vi "PositionSave_MD.vi"() -> ()   [LabVIEW 2012]
doc: "<b>Description</b>\n-------------\nThis is the Main VI for the Position Save Module and has a UI.\n\nThe module has a dependency with the main Sci-Scan software as it listens for events using the GFG."
uses:
  Custom Control and Typedefs/ChannelSelector_for_PosSave.ctl
  Custom Controls/PositionSaveMod.ctl
  Custom Control and Typedefs/Overlay Control.ctl
  SubVIs/PositionSaveFGVCommands.ctl
  Custom Control and Typedefs/UI Controls Refnum.ctl
  <vilib>/vision/Image Controls.llb/IMAQ Image.ctl
  Custom Control and Typedefs/ImageCluster.ctl
  SubVIs/Chnl_2_tab_Commands.ctl
  SubVIs/Image Validity FGV_Commands.ctl
  Custom Controls/MAIN Image panel tab Control type def.ctl
  CommonResource VIs/UI Control and Indicator properties_Commands.ctl
  CommonResource VIs/FormatTableStyle_Commands.ctl
  Custom Control and Typedefs/PositionData.ctl
  SubVIs/ImageIO_commands.ctl
  GFG/GFG library.lvlib
panel:
  in  "FOCUS2":bool
  in  "Overlay Controls":T1={"auto scale\n      Red "=TRUE, "Min Max Saved (Green)"={0.0, 1618.0}, "auto scale\n      Green"=TRUE, "Min Max Saved (Red)"={0.0, 1618.0}} {"Min Max Saved (Red)" scale=-100.0..2047.0; "Min Max Saved (Green)" scale=-100.0..2047.0}
  in  "Hide":T2
  in  "Copy Button":bool
  out "File Path":path
  in  "Overlay":bool
  in  "Table Navigation Cluster":T3
  in  "Vert_Cluster":T4
  in  "Big_Table":string[][](table)
  in  "Notes_Table":string[][](table)
  in  "Source":T5
  in  "step.size.z 2":u16(ring)=6 items=["  1"=1, "  2"=2, "  5"=5, " 10"=10, " 20"=20, " 50"=50, "100"=100]
  in  "Stage Stop 2":bool
  in  "Z UP 2":bool
  in  "Z DOWN 2":bool
  out "String 26":string
  in  "step.size.xy 2":u16(ring)=6 items=["  1"=1, "  2"=2, "  5"=5, " 10"=10, " 20"=20, " 50"=50, "100"=100]
  in  "Y UP 2":bool
  in  "X LEFT 2":bool
  in  "Y DOWN 2":bool
  in  "X RIGHT 2":bool
  out "String 25":string
  in  "setY 2":dbl caption="Z-Stepper" format="%#.1f"
  in  "setX 2":dbl caption="Z-Stepper" format="%#.1f"
  in  "setZ 2":dbl caption="set" format="%#.1f"
  out "String 24":string
  out "posZ 2":dbl caption="actual" format="%#.1f"
  out "posX 2":dbl caption="Z-Stepper" format="%#.1f"
  out "posY 2":dbl caption="Z-Stepper" format="%#.1f"
  out "String 23":string
  in  "Hor_Cluster":T6
  out "XY Graph":cluster{dbl[], dbl[]}[](graph)
  out "Saved Image":T7(plugin-control)
  out "Current Image":T7(plugin-control)
  # "current pos."
  # "go to pos."
  # "Red (Current Image)"
  # "Green (Saved Image)"
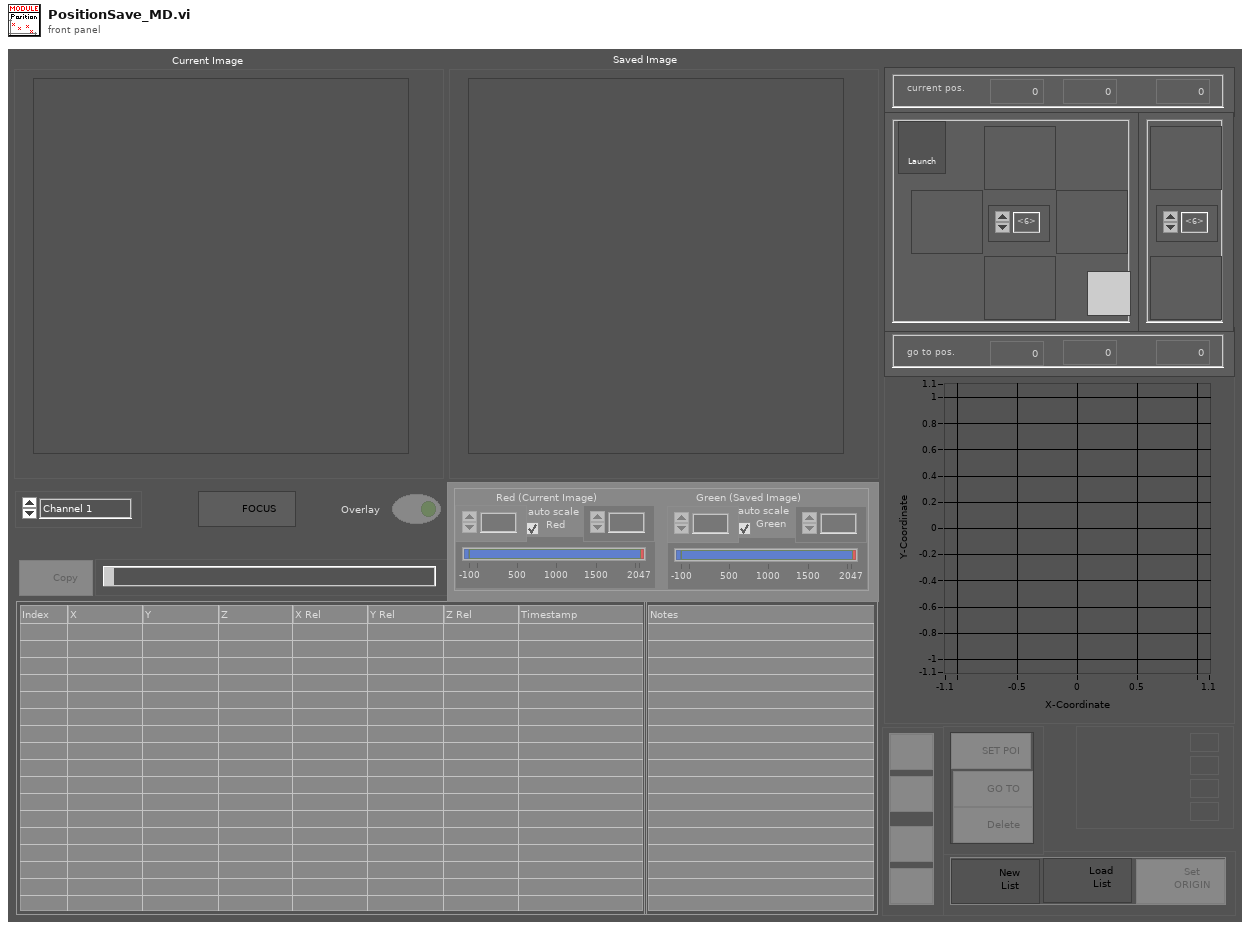
[diagram p1: front panel]
types:
  T1 = typedef "Overlay Control.ctl" = cluster{"auto scale\n      Red ":bool, "Min Max Saved (Green)":cluster{dbl, dbl}, "auto scale\n      Green":bool, "Min Max Saved (Red)":cluster{dbl, dbl}}
  T2 = typedef "PositionSaveMod.ctl" = bool
  T3 = cluster{"Table Index Up":bool, "Table Index Up-End":bool, "Table Index Down":bool, "Table Index Down-End":bool}
  T4 = cluster{"Delete item":bool, "SET POI":bool, "GO TO":bool}
  T5 = typedef "ChannelSelector_for_PosSave.ctl" = enum16{"Channel 1", "Channel 2", "Channel 3", "Channel 4"}
  T6 = cluster{"New List":bool, "Load List":bool, "Set new Origin":bool}
  T7 = typedef "IMAQ Image.ctl" = refnum<image>
  T8 = typedef "Image Type" = u32
  T9 = typedef "UI Controls Refnum.ctl" = cluster{"GO TO":refnum<vi>, "Load List":refnum<vi>, "Big Table":refnum<vi>, "Notes Table":refnum<vi>, "New List":refnum<vi>, "Delete Item":refnum<vi>, "Set New Origin":refnum<vi>, "Set POI":refnum<vi>, "Saved Image":refnum<vi>, "Current Image":refnum<vi>, "step.size.xy 2":refnum<vi>, "step.size.z 2":refnum<vi>, "Source":refnum<vi>, "Table Up-End":refnum<vi>, "Table Up":refnum<vi>, "Table Down":refnum<vi>, "Table Down-End":refnum<vi>, "Copy Button":refnum<vi>, "Hide":refnum<vi>, "Overlay Controls":refnum<vi>, "Overlay":refnum<vi>, "XYGraph":refnum<vi>, "FOCUS2":refnum<vi>}
  T10 = typedef "PositionSaveFGVCommands.ctl" = enum16{"Initialize", "NewList", "LoadList", "CopyList", "DeleteSelected", "SetPosition", "SetNewOrigin", "UpdateEntireTable", "GetPosition", "Shutdown and Cleanup"}
  T11 = typedef "ImageCluster.ctl" = cluster{"CurrentImage":T7, "SavedImage":T7}
  T12 = enum32{"Invalid", "Standard", "Closed", "Hidden", "Minimized", "Maximized"}
  T13 = typedef "Image Validity FGV_Commands.ctl" = enum16{"Set validity status", "Get Validity status"}
  T14 = typedef "Chnl_2_tab_Commands.ctl" = enum16{"ChannelToTab", "TabToChannel"}
  T15 = typedef "UI Control and Indicator properties_Commands.ctl" = enum16{"Enable", "Disable", "Disable and Grey", "Make Visible", "Make Invisible"}
  T16 = typedef "MAIN Image panel tab Control type def.ctl" = enum32{"Channel 1", "Channel 2", "Channel 3", "Channel 4", "all channels", "RGB overlay", "ROI", "arbitrary line scan"}
  T17 = cluster{"moveXabs":dbl, "moveYabs":dbl, "moveZabs":dbl}
  T18 = typedef "FormatTableStyle_Commands.ctl" = enum16{"Colour Row", "Uncolour Row", "Bold Row", "Clear table", "UpdateVisibleRows"}
  T19 = typedef "PositionData.ctl" = cluster{"X":dbl, "Y":dbl, "Z":dbl, "Base Path":path}
  T20 = typedef "ImageIO_commands.ctl" = enum16{"ReadImage", "WriteImage"}
  T21 = cluster{"WaveformChartRef":refnum<vi>, "DigitalRef":refnum<vi>, "ArrayRef":refnum<vi>, "TabControlRef":refnum<vi>, "EnumRef":refnum<vi>, "RingRef":refnum<vi>, "BooleanRef":refnum<vi>, "KnobRef":refnum<vi>, "SlideRef":refnum<vi>, "PathRef":refnum<vi>, "StringRef":refnum<vi>, "ComboBox":refnum<vi>, "WaveformGraphRef":refnum<vi>}
  T22 = typedef "LVRowAndColumnTypeDef.ctl" = cluster{"Row":i32, "Column":i32}
  T23 = typedef "eventvkey.ctl" = enum16{"ASCII", "Enter", "Return", "Shift", "Ctrl", "Alt", "Cmd", "Opt", "Caps", "NumLock", "Clear", "Break", "Up", "Down", "Left", "Right", "Insert", "Delete", "Home", "End", "PageUp", "PageDown", "Escape", "Help", "Pause", "ScrollLock", "F1", "F2", "F3", "F4", "F5", "F6", "F7", "F8", "F9", "F10", "F11", "F12", "F13", "F14", "F15", "F16", "F17", "F18", "F19", "F20", "F21", "F22", "F23", "F24", "Play", "VolumeUp", "VolumeDown", "Mute", "Two Byte Char"}
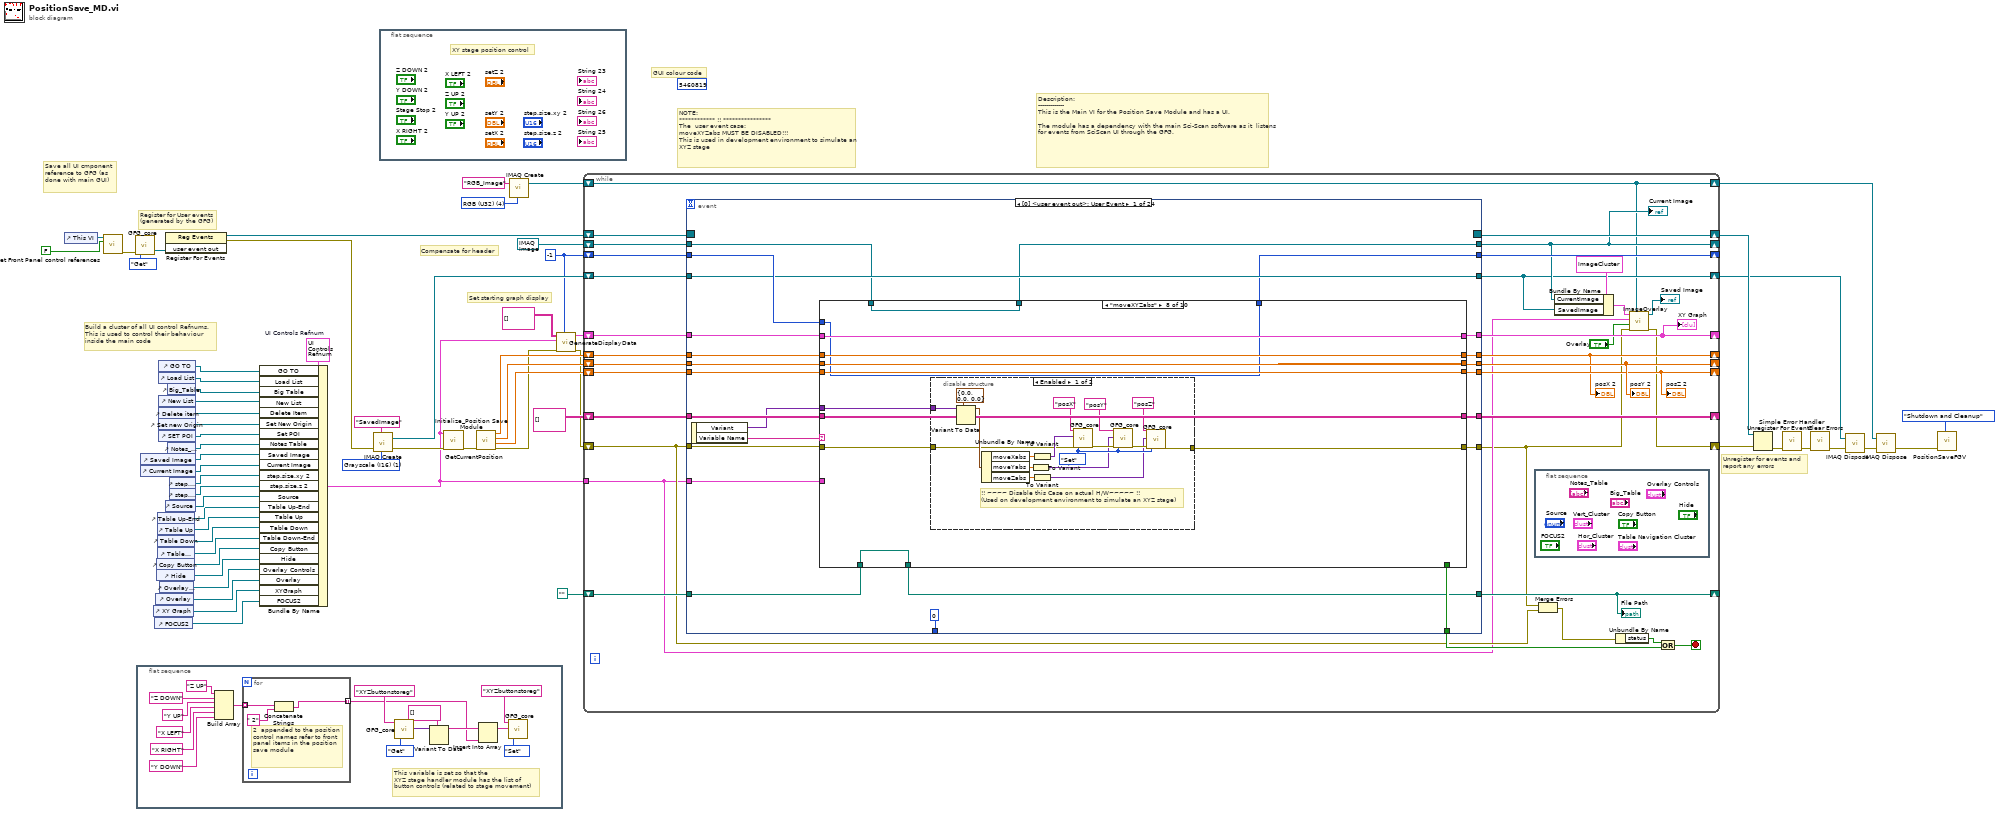
[diagram p0: block diagram]
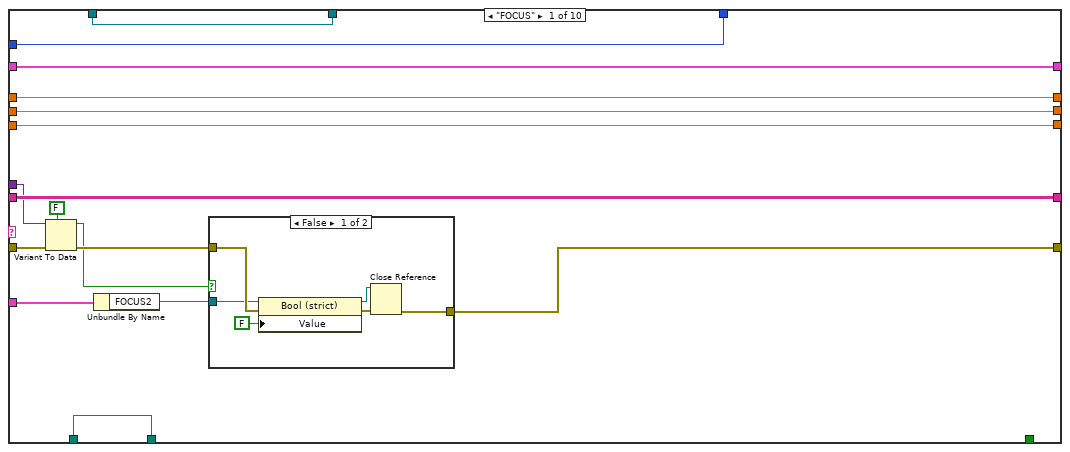
[diagram p2: hidden frame]
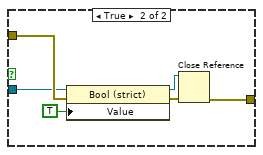
[diagram p3: hidden frame]
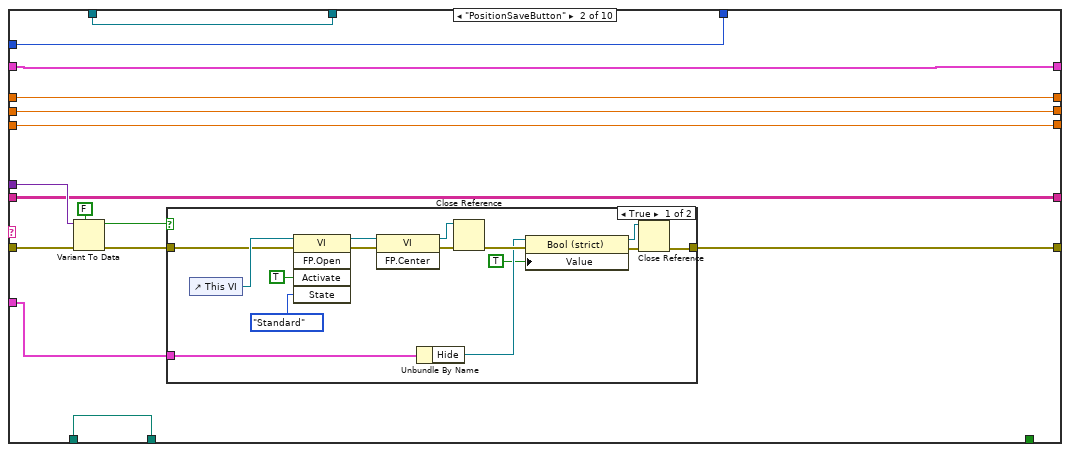
[diagram p4: hidden frame]
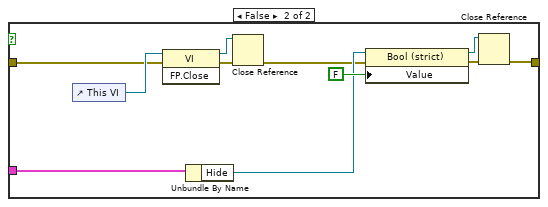
[diagram p5: hidden frame]
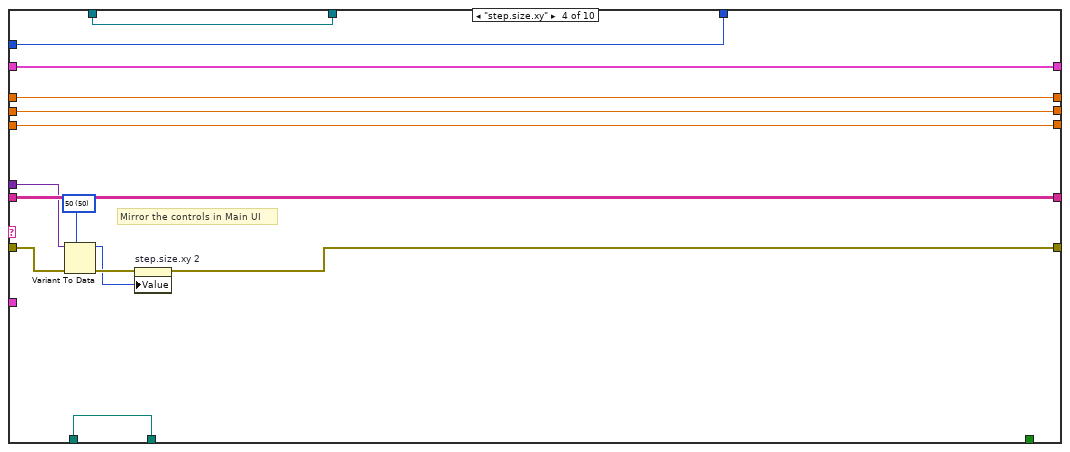
[diagram p7: hidden frame]
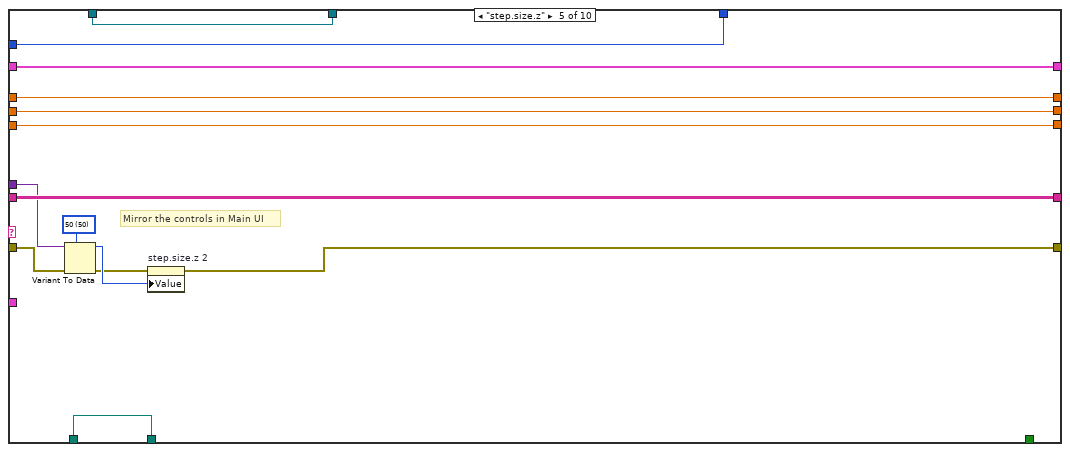
[diagram p8: hidden frame]
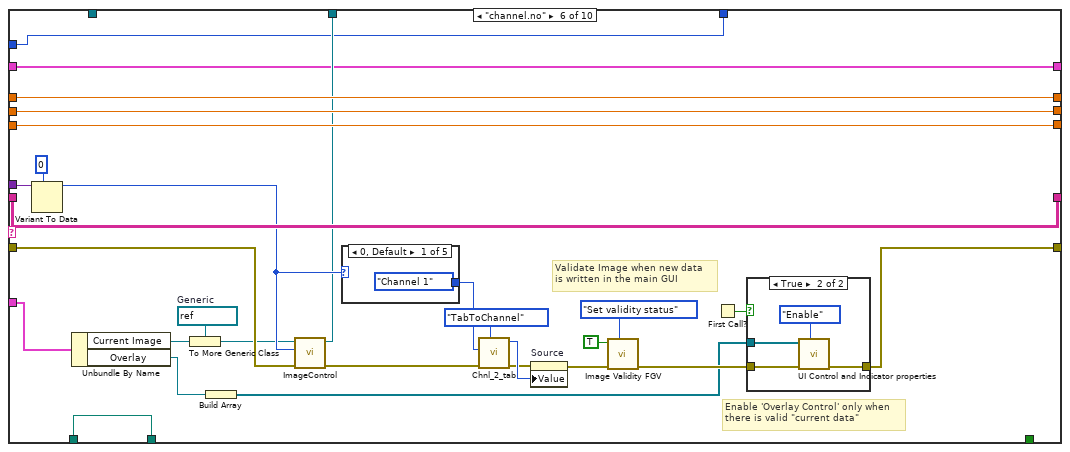
[diagram p9: hidden frame]
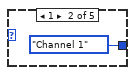
[diagram p11: hidden frame]
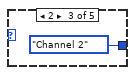
[diagram p12: hidden frame]
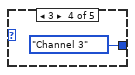
[diagram p13: hidden frame]
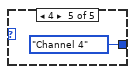
[diagram p14: hidden frame]
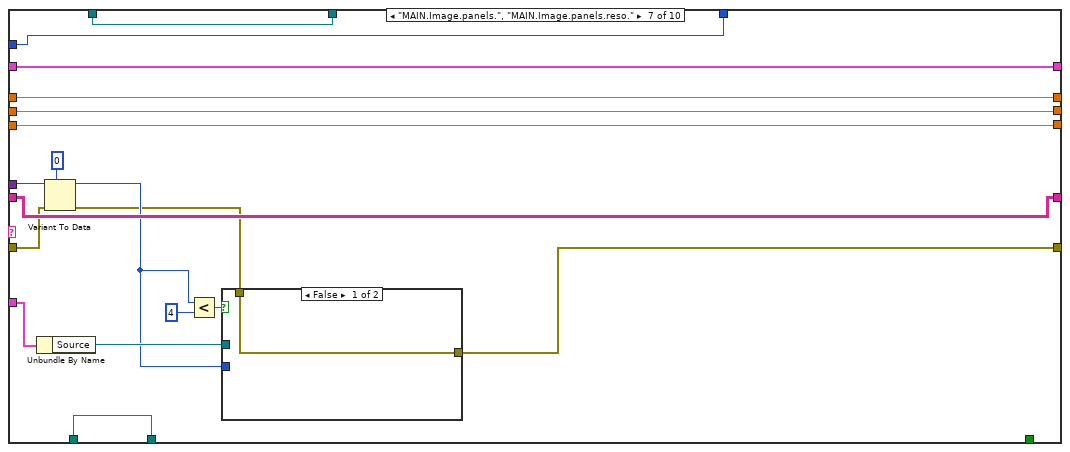
[diagram p15: hidden frame]
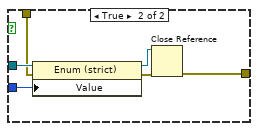
[diagram p16: hidden frame]
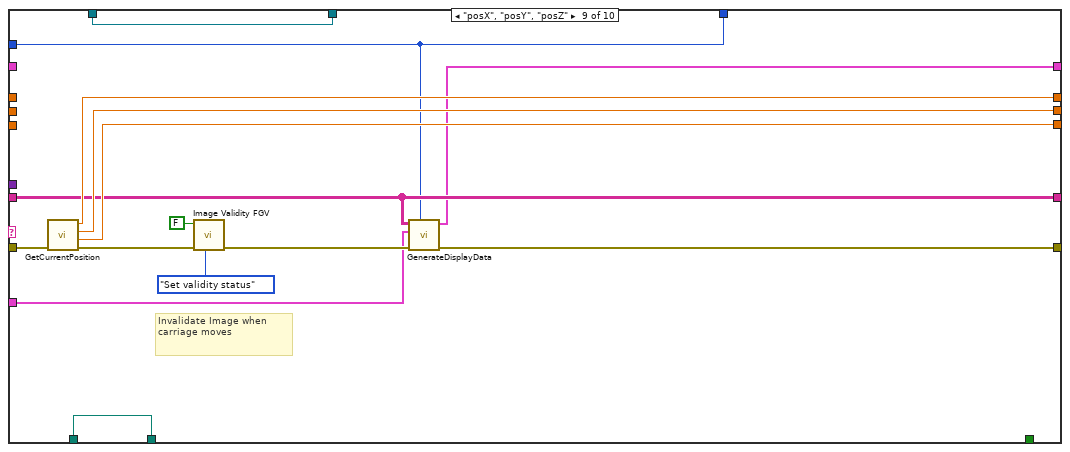
[diagram p18: hidden frame]
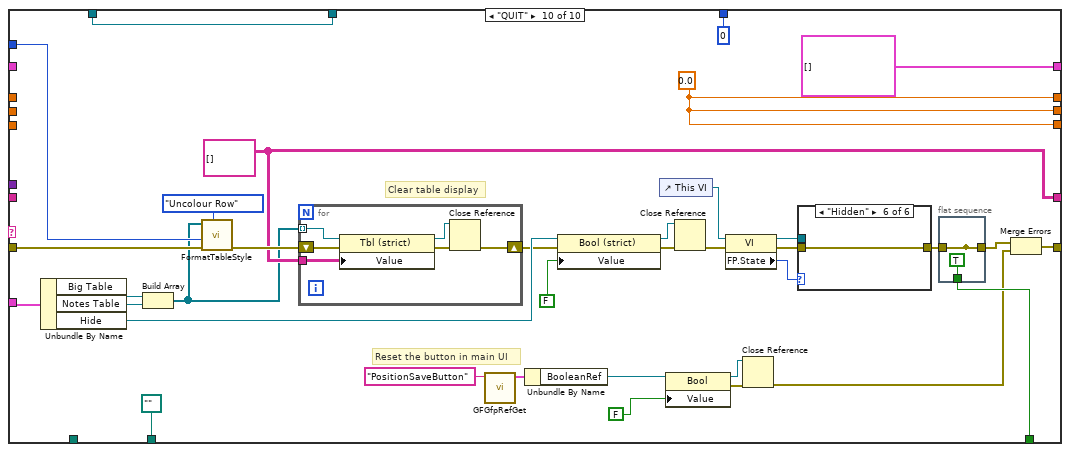
[diagram p19: hidden frame]
diagram:
  w17 = T8 4 items=["Grayscale (U8)", "Grayscale (I16)", "Grayscale (SGL)", "Complex (CSG)", "RGB (U32)", "HSL (U32)", "RGB (U64)", "Grayscale (U16)"] ("Image Type")
  w28 = T8 1 items=["Grayscale (U8)", "Grayscale (I16)", "Grayscale (SGL)", "Complex (CSG)", "RGB (U32)", "HSL (U32)", "RGB (U64)", "Grayscale (U16)"] ("Image Type")
  (unwired) u32 5460819 ("Active Cell:Cell Background Color")
  w9 = -1
  w53 = T9 {"GO TO"=refnum, "Load List"=refnum, "Big Table"=refnum, "Notes Table"=refnum, "New List"=refnum, "Delete Item"=refnum, "Set New Origin"=refnum, "Set POI"=refnum, "Saved Image"=refnum, "Current Image"=refnum, "step.size.xy 2"=refnum, "step.size.z 2"=refnum, "Source"=refnum, "Table Up-End"=refnum, "Table Up"=refnum, "Table Down"=refnum, "Table Down-End"=refnum, "Copy Button"=refnum, "Hide"=refnum, "Overlay Controls"=refnum, "Overlay"=refnum, "XYGraph"=refnum, "FOCUS2"=refnum}  # UI Controls Refnum
  # "Set starting graph display"
  # "Compensate for header"
  # "GUI colour code"
  # "Save all UI cmponent reference to GFG (as done with main GUI)"
  # "NOTE:\n************ !! ****************\nThe  user event case:\nmoveXYZabs MUST BE DISABLED!!!\nThis is used in development environment to simulate an XYZ stage"
  # "Register for User events\n(generated by the GFG)"
  # "Build a cluster of all UI control Refnums.\nThis is used to control their behaviour \ninside the main code"
  # "Unregister for events and \nreport any errors"
  # "Description:\n-------------\nThis is the Main VI for the Position Save Module and has a UI.\n\nThe module has a dependency with the main Sci-Scan software as it  listens for events from SciScan UI through the GFG."
  n1 = control-ref of="This VI"() -> (w46:refnum<vi>)
  n2 = call "get Front Panel control references.vi"("Signalling (Default: T)"=FALSE, "Main VI"=w46) -> ("error out"=w45:errorcluster)  [unwired: 9 in]
  n3 = call "GFG_core.vi"("error in (no error)"=w45, "Action"=enum16{"Init", "Set", "Get"}."Get") -> ("user event out"=w59:refnum<user-event>)  [unwired: 11 in, 6 out]
  n4 = flat-sequence {
    frame #0 {
      # "This variable is set so that the \nXYZ stage handler module has the list of\nbutton controls (related to stage movement)"
      n5 = Build Array("Z UP" ("Variable Name in"), "Z DOWN" ("Variable Name in"), "Y UP" ("Variable Name in"), "X LEFT" ("Variable Name in"), "X RIGHT" ("Variable Name in"), "Y DOWN" ("Variable Name in")) -> (w71:string[])
      n6 = for {
        tunnel: w71 -> [w80] mode=indexing
        tunnel: [w78] -> w62 mode=indexing
        # "2  appended to the position control names refer to front panel items in the position save module"
        n7 = Concatenate Strings(w80, " 2" ("string")) -> (w78:string)
      }
      n8 = call "GFG_core.vi"("Variable Name in"="XYZbuttonstoreg", "Action"=enum16{"Init", "Set", "Get"}."Get") -> ("Variant Out"=w65:variant)  [unwired: 11 in, 6 out]
      n9 = Variant To Data(type=string[] [], Variant=w65) -> (data=w63:string[])  [unwired: 1 in, 1 out]
      n10 = Insert Into Array(array=w63, new element=w62) -> (w64:string[])  [unwired: 1 in]
      n11 = call "GFG_core.vi"("Variable Name in"="XYZbuttonstoreg", "Variant in"=w64, "Action"=enum16{"Init", "Set", "Get"}."Set") -> ()  [unwired: 10 in, 7 out]
    }
  }
  n12 = control-ref of="Saved Image"() -> (w41:refnum<vi>)
  n13 = control-ref of="Current Image"() -> (w40:refnum<vi>)
  n14 = control-ref of="XY Graph"() -> (w13:refnum<vi>)
  n15 = control-ref of="FOCUS2"() -> (w7:refnum<vi>)
  n16 = control-ref of="Overlay"() -> (w14:refnum<vi>)
  n17 = control-ref of="Copy Button"() -> (w26:refnum<vi>)
  n18 = control-ref of="Hide"() -> (w22:refnum<vi>)
  n19 = control-ref of="Table Up-End"() -> (w35:refnum<vi>)
  n20 = control-ref of="Table Up"() -> (w34:refnum<vi>)
  n21 = control-ref of="Table Down"() -> (w33:refnum<vi>)
  n22 = control-ref of="Table Down-End"() -> (w32:refnum<vi>)
  n23 = control-ref of="GO TO"() -> (w52:refnum<vi>)
  n24 = control-ref of="Load List"() -> (w51:refnum<vi>)
  n25 = control-ref of="New List"() -> (w50:refnum<vi>)
  n26 = control-ref of="Delete item"() -> (w49:refnum<vi>)
  n27 = control-ref of="Set new Origin"() -> (w48:refnum<vi>)
  n28 = control-ref of="SET POI"() -> (w47:refnum<vi>)
  n29 = control-ref of="Overlay Controls"() -> (w19:refnum<vi>)
  n30 = control-ref of="Source"() -> (w37:refnum<vi>)
  n31 = register-events(w59) -> (reference out=w60:refnum<event-registration>, error out=w8:errorcluster)  [unwired: 2 in]
  n32 = control-ref of="Big_Table"() -> (w31:refnum<vi>)
  n33 = control-ref of="Notes_Table"() -> (w43:refnum<vi>)
  n34 = control-ref of="step.size.xy 2"() -> (w39:refnum<vi>)
  n35 = control-ref of="step.size.z 2"() -> (w38:refnum<vi>)
  n36 = Bundle By Name(cluster=w53, "GO TO"=w52, "Load List"=w51, "Big Table"=w31, "New List"=w50, "Delete Item"=w49, "Set New Origin"=w48, "Set POI"=w47, "Notes Table"=w43, "Saved Image"=w41, "Current Image"=w40, "step.size.xy 2"=w39, "step.size.z 2"=w38, "Source"=w37, "Table Up-End"=w35, "Table Up"=w34, "Table Down"=w33, "Table Down-End"=w32, "Copy Button"=w26, "Hide"=w22, "Overlay Controls"=w19, "Overlay"=w14, "XYGraph"=w13, "FOCUS2"=w7) -> (w12:T9)
  n37 = call "IMAQ Create"("Image Name"="SavedImage", "Image Type"=w28, "error in (no error)"=w8) -> ("New Image"=w27:T7, "error out"=w29:errorcluster)  [unwired: 2 in]
  n38 = flat-sequence {
    frame #0 {
      # "XY stage position control"
    }
  }
  n39 = call "Initialize_Position Save Module.vi"("Error In"=w29, "UI Controls Refnum"=w12) -> ("Error Out"=w36:errorcluster)  [unwired: 9 in]
  n40 = call "GetCurrentPosition.vi"("Error In"=w36) -> ("Error Out"=w11:errorcluster, "Z"=w56:dbl, "Y"=w57:dbl, "X"=w58:dbl)  [unwired: 7 in]
  n41 = call "IMAQ Create"("Image Name"="RGB_Image", "Image Type"=w17) -> ("New Image"=w16:T7)  [unwired: 3 in, 1 out]
  n42 = call "GenerateDisplayData.vi"("Index"=w9, "Error In"=w11, "UI Controls Refnum"=w12, "2D Data IN"=string[][] []) -> ("Error Out"=w10:errorcluster, "Plot Data OUT"=w20:cluster{dbl[], dbl[]}[])  [unwired: 4 in, 2 out]
  n43 = while {
    shift-right: [w81] -> w24
    shift-left: w10 -> [w92]
    shift-right: [w109] -> w54
    shift-left: w60 -> [w110]
    shift-right: [w94] -> _
    shift-left: w58 -> [w108]
    shift-right: [w103] -> _
    shift-left: w57 -> [w107]
    shift-right: [w102] -> _
    shift-left: w56 -> [w106]
    shift-right: [w93] -> _
    shift-left: w20 -> [w105]
    shift-right: [w100] -> _
    shift-left: string[][] [] ("Formatted Table Data") -> [w104]
    tunnel: w12 -> [w90]
    shift-right: [w88] -> _
    shift-left: T7 refnum ("Saved Image OUT") -> [w101]
    shift-right: [w98] -> _
    shift-left: w9 -> [w99]
    shift-right: [w87] -> w3
    shift-left: w27 -> [w97]
    shift-right: [w95] -> _
    shift-left: path "" -> [w96]
    shift-right: [w84] -> w2
    shift-left: w16 -> [w84]
    stop <- w111 stop-if-true
    n44 = event shown="[0] <user event out>: User Event" {
      selector: w110 -> [_ _ _ _ _ _ _ _ _ _ _ _ _ _ _ _ _ _ _ _ _ _ _ _]
      dyn-events: [_ _ _ _ _ _ _ _ _ _ _ _ _ _ _ _ _ _ _ _ _ _ _ _] -> w109
      timeout: _ -> [_ _ _ _ _ _ _ _ _ _ _ _ _ _ _ _ _ _ _ _ _ _ _ _]
      tunnel: [w137 _ _ _ _ _ _ _ _ _ _ _ _ _ _ _ _ _ _ _ _ _ _ FALSE] -> w113
      tunnel: w108 -> [w133 w426 w447 w480 w540 w604 w715 w786 w879 w982 w1033 w1070 w1093 w1145 w1193 w1242 w1286 w1333 w1354 w1373 w1392 w1451 w1474 w1480]
      tunnel: w107 -> [w132 w425 w446 w479 w539 w603 w714 w787 w878 w981 w1032 w1069 w1092 w1144 w1192 w1241 w1285 w1332 w1353 w1372 w1391 w1450 w1473 w1479]
      tunnel: w106 -> [w131 w424 w445 w478 w538 w591 w713 w788 w877 w980 w1031 w1068 w1091 w1143 w1191 w1240 w1284 w1331 w1352 w1371 w1390 w1449 w1472 w1478]
      tunnel: [w134 w426 w447 w480 w540 w592 w715 w786 w879 w982 w1033 w1070 w1093 w1145 w1193 w1242 w1286 w1333 w1354 w1373 w1392 w1451 w1474 w1480] -> w94
      tunnel: [w135 w425 w446 w479 w539 w590 w714 w787 w878 w981 w1032 w1069 w1092 w1144 w1192 w1241 w1285 w1332 w1353 w1372 w1391 w1450 w1473 w1479] -> w103
      tunnel: [w136 w424 w445 w478 w538 w589 w713 w788 w877 w980 w1031 w1068 w1091 w1143 w1191 w1240 w1284 w1331 w1352 w1371 w1390 w1449 w1472 w1478] -> w102
      tunnel: [w122 w423 w444 w457 w522 w597 w706 w762 w870 w956 w1005 w1067 w1090 w1121 w1169 w1220 w1266 w1330 w1351 w1370 w1375 w1448 w1471 w1477] -> w93
      tunnel: w105 -> [w123 w423 w444 _ _ w598 w705 _ w869 _ _ w1067 w1090 _ _ _ _ w1330 w1351 w1370 _ w1448 w1471 w1477]
      tunnel: [w129 w419 w440 w459 w523 w602 w707 w765 w874 w957 w1006 w1058 w1088 w1124 w1171 w1222 w1268 w1329 w1347 w1369 w1379 w1443 w1467 w1481] -> w100
      tunnel: w92 -> [w130 w414 w438 w475 w535 w588 w710 w778 w875 w978 w1029 w1063 w1081 w1138 w1186 w1237 w1279 w1327 w1346 w1359 w1384 w1444 w1466 w1483]
      tunnel: [w128 w413 w438 w449 w521 w601 w708 w767 w871 w954 w1007 w1059 w1086 w1123 w1173 w1224 w1270 w1313 w1345 w1356 w1376 w1444 w1465 w1487] -> w82
      tunnel: w104 -> [w127 w419 w440 w472 w532 w584 w702 w779 w876 w957 w1006 w1058 w1085 w1124 w1171 w1222 w1268 w1329 w1347 w1369 w1379 w1443 w1467 w1481]
      tunnel: w90 -> [w124 w416 _ w450 w519 w579 w703 w763 w872 w953 w1004 w1065 w1073 w1122 w1170 w1221 w1267 _ _ _ w1378 _ _ _]
      tunnel: [w120 w422 w443 w469 w529 w594 w698 w782 w865 w962 w1014 w1066 w1089 w1130 w1178 w1218 w1275 w1324 w1343 w1368 w1386 w1447 w1463 w1485] -> w88
      tunnel: w101 -> [w116 w422 w443 w469 w529 w594 w698 w782 w865 w962 w1014 w1066 w1089 w1130 w1178 w1218 w1275 w1324 w1343 w1368 w1386 w1447 w1463 w1485]
      tunnel: w99 -> [w125 w421 w442 w471 w531 w600 w701 w785 w868 w975 w1026 w1057 w1072 w1135 w1185 w1236 w1278 w1323 w1342 w1367 w1383 w1440 w1462 w1484]
      tunnel: [w117 w421 w442 w458 w520 w599 w700 w764 w873 w955 w1009 w1057 w1072 w1126 w1172 w1223 w1269 w1323 w1342 w1367 w1377 w1440 w1462 w1484] -> w98
      tunnel: [w121 w420 w441 w466 w527 w576 w695 w784 w863 w960 w1012 w1056 w1080 w1128 w1176 w1219 w1273 w1322 w1341 w1366 w1381 w1446 w1461 w1486] -> w87
      tunnel: w97 -> [w121 w420 w441 w468 w530 w595 w697 w781 w866 w963 w1015 w1056 w1080 w1131 w1179 w1228 w1276 w1322 w1341 w1366 w1382 w1446 w1461 w1486]
      tunnel: [w118 w418 w439 w465 w525 w578 w694 w774 w861 w959 w1011 w1055 w1079 w1127 w1175 w1226 w1272 w1318 w1340 w1365 w1389 w1445 w1460 w1476] -> w95
      tunnel: w96 -> [w119 w418 w439 _ _ w577 _ w773 w860 w959 w1011 w1055 w1079 w1127 w1175 w1226 w1272 w1318 w1340 w1365 w1389 w1445 w1460 w1476]
      tunnel: [0 ("x-y 2") 1 ("x-y 2") 2 ("x-y 2") 3 ("x-y 2") 4 ("x-y 2") 5 ("x-y 2") 6 ("x-y 2") 7 ("x-y 2") 8 ("x-y 2") 9 ("x-y 2") 10 ("x-y 2") 11 ("x-y 2") 12 ("x-y 2") 13 ("x-y 2") 14 ("x-y 2") 15 ("x-y 2") 16 ("x-y 2") 17 ("x-y 2") 18 ("x-y 2") 19 ("x-y 2") 20 ("x-y 2") 21 ("x-y 2") 22 ("x-y 2") 23 ("x-y 2")] -> _
      event User Event {
        n45 = event-data() -> ("Variant"=w126:variant, "Variable Name"=w114:string)  [unwired: 1 in]
        n46 = case shown="\"moveXYZabs\"" w114 {
          tunnel: [_ _ _ _ _ _ _ _ _ w355] -> w137
          tunnel: [w151 w178 w209 w227 w241 w270 w298 w316 w351 w385] -> w136
          tunnel: [w152 w179 w210 w228 w242 w271 w299 w317 w350 w385] -> w135
          tunnel: [w153 w180 w211 w229 w243 w272 w300 w318 w349 w385] -> w134
          tunnel: w133 -> [w153 w180 w211 w229 w243 w272 w300 w318 _ _]
          tunnel: w132 -> [w152 w179 w210 w228 w242 w271 w299 w317 _ _]
          tunnel: w131 -> [w151 w178 w209 w227 w241 w270 w298 w316 _ _]
          tunnel: w130 -> [w144 w177 w207 w224 w238 w260 w291 w312 w348 w382]
          tunnel: [w150 w171 w208 w226 w240 w269 w297 w313 w342 w379] -> w129
          tunnel: [w140 w172 w207 w221 w235 w246 w288 w314 w343 w354] -> w128
          tunnel: w127 -> [w150 w171 w208 w226 w240 w269 w297 w313 w342 _]
          tunnel: w126 -> [w142 w175 _ w220 w234 w268 w296 w315 _ _]
          tunnel: [w146 w166 w215 w216 w230 w259 w292 w308 w338 w362] -> w120
          tunnel: w125 -> [w147 w168 w212 w217 w231 w249 w293 w309 w337 w384]
          tunnel: w124 -> [w139 w167 _ _ _ w254 w290 _ w339 w383]
          tunnel: w123 -> [w149 w169 w214 w219 w233 w258 w295 w311 _ _]
          tunnel: [w149 w169 w214 w219 w233 w258 w295 w311 w341 cluster{dbl[], dbl[]}[] [] ("Plot Data OUT")] -> w122
          tunnel: w119 -> [w148 w170 w213 w218 w232 w250 w294 w310 w340 _]
          tunnel: [w148 w170 w213 w218 w232 w250 w294 w310 w340 path ""] -> w118
          tunnel: [w147 w168 w212 w217 w231 w249 w293 w309 w337 0 ("Row")] -> w117
          tunnel: w116 -> [w146 w166 w215 w216 w230 _ w292 w308 w338 w362]
          frame "FOCUS" {
            n47 = Variant To Data(error in=w144, type=FALSE ("Value"), Variant=w142) -> (data=w141:bool, error out=w143:errorcluster)
            n48 = Unbundle By Name(w139) -> ("FOCUS2"=w138:refnum<vi>)
            n49 = case shown="False" w141 {
              tunnel: w143 -> [w158 w164]
              tunnel: [w155 w161] -> w140
              tunnel: w138 -> [w154 w160]
              frame False {
                n50 = property class="Bool (strict)"(reference=w154, error in=w158, "Value"=FALSE) -> (reference out=w156:refnum<vi>, error out=w157:errorcluster)
                n51 = Close Reference(reference=w156, error in (no error)=w157) -> (error out=w155:errorcluster)
              }
              frame True {
                n52 = property class="Bool (strict)"(reference=w160, error in=w164, "Value"=TRUE) -> (reference out=w162:refnum<vi>, error out=w163:errorcluster)
                n53 = Close Reference(reference=w162, error in (no error)=w163) -> (error out=w161:errorcluster)
              }
            }
          }
          frame "PositionSaveButton" {
            n54 = Variant To Data(error in=w177, type=FALSE, Variant=w175) -> (data=w173:bool, error out=w174:errorcluster)
            n55 = case shown="True" w173 {
              tunnel: w174 -> [w194 w205]
              tunnel: [w181 w199] -> w172
              tunnel: w167 -> [w186 w198]
              frame True {
                n56 = control-ref of="This VI"() -> (w195:refnum<vi>)
                n57 = invoke class="VI" method="FP.Open"(reference=w195, error in=w194, "Activate"=TRUE ("Activate?"), "State"=T12."Standard") -> (reference out=w191:refnum<vi>, error out=w190:errorcluster)  [unwired: 1 in, 3 out]
                n58 = invoke class="VI" method="FP.Center"(reference=w191, error in=w190) -> (reference out=w188:refnum<vi>, error out=w189:errorcluster)  [unwired: 1 in, 1 out]
                n59 = Unbundle By Name(w186) -> ("Hide"=w185:refnum<vi>)
                n60 = Close Reference(reference=w188, error in (no error)=w189) -> (error out=w187:errorcluster)
                n61 = property class="Bool (strict)"(reference=w185, error in=w187, "Value"=T2 TRUE) -> (reference out=w182:refnum<vi>, error out=w183:errorcluster)
                n62 = Close Reference(reference=w182, error in (no error)=w183) -> (error out=w181:errorcluster)
              }
              frame False {
                n63 = control-ref of="This VI"() -> (w206:refnum<vi>)
                n64 = invoke class="VI" method="FP.Close"(reference=w206, error in=w205) -> (reference out=w203:refnum<vi>, error out=w204:errorcluster)  [unwired: 1 in, 1 out]
                n65 = Unbundle By Name(w198) -> ("Hide"=w197:refnum<vi>)
                n66 = Close Reference(reference=w203, error in (no error)=w204) -> (error out=w196:errorcluster)
                n67 = property class="Bool (strict)"(reference=w197, error in=w196, "Value"=T2 FALSE) -> (reference out=w200:refnum<vi>, error out=w201:errorcluster)
                n68 = Close Reference(reference=w200, error in (no error)=w201) -> (error out=w199:errorcluster)
              }
            }
          }
          frame Default {
          }
          frame "step.size.xy" {
            w225 = u16 50 items=["  1"=1, "  2"=2, "  5"=5, " 10"=10, " 20"=20, " 50"=50, "100"=100] ("step.size.xy 2")
            # "Mirror the controls in Main UI"
            n69 = Variant To Data(error in=w224, type=w225, Variant=w220) -> (data=w222:u16, error out=w223:errorcluster)
            n70 = property on="step.size.xy 2" class="Ring (strict)"(error in=w223, "Value"=w222) -> (error out=w221:errorcluster)  [unwired: 1 in, 1 out]
          }
          frame "step.size.z" {
            w239 = u16 50 items=["  1"=1, "  2"=2, "  5"=5, " 10"=10, " 20"=20, " 50"=50, "100"=100] ("step.size.xy 2")
            # "Mirror the controls in Main UI"
            n71 = Variant To Data(error in=w238, type=w239, Variant=w234) -> (data=w237:u16, error out=w236:errorcluster)
            n72 = property on="step.size.z 2" class="Ring (strict)"(error in=w236, "Value"=w237) -> (error out=w235:errorcluster)  [unwired: 1 in, 1 out]
          }
          frame "channel.no" {
            w253 = refnum<vi> refnum  # Generic
            # "Enable 'Overlay Control' only when there is valid \"current data\""
            # "Validate Image when new data\nis written in the main GUI"
            n73 = Variant To Data(type=0, Variant=w268) -> (data=w266:i32)  [unwired: 1 in, 1 out]
            n74 = Unbundle By Name(w254) -> ("Current Image"=w252:refnum<vi>, "Overlay"=w244:refnum<vi>)
            n75 = To More Generic Class(target class=w253, reference=w252) -> (generic class reference=w251:refnum<vi>)
            n76 = Build Array(w244) -> (w245:refnum<vi>[])
            n77 = call "ImageControl.vi"("Error In"=w260, "Channel No"=w266, "Image Refnum (Generic)"=w251) -> ("Error Out"=w262:errorcluster, "Current Image"=w259:T7)  [unwired: 7 in]
            n78 = case shown="0, Default" w266 {
              tunnel: [MAIN_Image_panel_tab_Control_type_def."Channel 1" ("Tab IN") MAIN_Image_panel_tab_Control_type_def."Channel 1" ("Tab IN") MAIN_Image_panel_tab_Control_type_def."Channel 2" ("Tab IN") MAIN_Image_panel_tab_Control_type_def."Channel 3" ("Tab IN") MAIN_Image_panel_tab_Control_type_def."Channel 4" ("Tab IN")] -> w264
              frame 0, Default {
              }
              frame 1 {
              }
              frame 2 {
              }
              frame 3 {
              }
              frame 4 {
              }
            }
            n79 = call "Chnl_2_tab.vi"("Command"=Chnl_2_tab_Commands."TabToChannel", "Error In"=w262, "Tab IN"=w264) -> ("Error Out"=w261:errorcluster, "Channel  OUT"=w263:T5)  [unwired: 6 in, 1 out]
            n80 = property on="Source" class="Enum (strict)"(error in=w261, "Value"=w263) -> (error out=w255:errorcluster)  [unwired: 1 in, 1 out]
            n81 = call "Image Validity FGV.vi"("Image Validity FGV_Commands"=Image_Validity_FGV_Commands."Set validity status", "Error In"=w255, "Validity status IN"=TRUE) -> ("Error Out"=w247:errorcluster)  [unwired: 7 in, 1 out]
            n82 = First Call?() -> (First Call?: T/F=w248:bool)
            n83 = case shown="True" w248 {
              tunnel: w247 -> [w273 w276]
              tunnel: [w273 w275] -> w246
              tunnel: w245 -> [_ w274]
              frame False {
              }
              frame True {
                n84 = call "UI Control and Indicator properties.vi"("Enable Command"=UI_Control_and_Indicator_properties_Commands."Enable", "Error In"=w276, "Control Refnums"=w274) -> ("Error Out"=w275:errorcluster)  [unwired: 8 in]
              }
            }
          }
          frame "MAIN.Image.panels.", "MAIN.Image.panels.reso." {
            n85 = Unbundle By Name(w290) -> ("Source"=w289:refnum<vi>)
            n86 = Variant To Data(error in=w291, type=0, Variant=w296) -> (data=w285:i32, error out=w283:errorcluster)
            n87 = Less?(x=w285, y=4) -> (x < y?=w286:bool)
            n88 = case shown="False" w286 {
              tunnel: w289 -> [_ w307]
              tunnel: [w301 w304] -> w288
              tunnel: w285 -> [_ w303]
              tunnel: w283 -> [w301 w302]
              frame False {
              }
              frame True {
                n89 = property class="Enum (strict)"(reference=w307, error in=w302, "Value"=w303) -> (reference out=w305:refnum<vi>, error out=w306:errorcluster)
                n90 = Close Reference(reference=w305, error in (no error)=w306) -> (error out=w304:errorcluster)
              }
            }
          }
          frame "moveXYZabs" {
            n91 = disable-structure shown="Enabled" {
              disable-tunnel: w315 -> [w329 _]
              disable-tunnel: [w328 w336] -> w314
              disable-tunnel: w312 -> [w319 w336]
              frame Enabled {
                w334 = enum16{"Init", "Set", "Get"}."Set" ("Action")
                # "!! ~~~~ Disable this Case on actual H/W~~~~~ !!\n(Used on development environment to simulate an XYZ stage)"
                n92 = Variant To Data(type=T17 {"moveXabs"=0.0, "moveYabs"=0.0, "moveZabs"=0.0} ("output cluster"), Variant=w329) -> (data=w330:T17)  [unwired: 1 in, 1 out]
                n93 = Unbundle By Name(w330) -> ("moveXabs"=w325:dbl, "moveYabs"=w324:dbl, "moveZabs"=w323:dbl)
                n94 = To Variant(anything=w324) -> (Variant=w321:variant)
                n95 = To Variant(anything=w325) -> (Variant=w322:variant)
                n96 = To Variant(anything=w323) -> (Variant=w320:variant)
                n97 = call "GFG_core.vi"("Variable Name in"="posX", "Variant in"=w322, "error in (no error)"=w319, "Action"=w334) -> ("error out"=w326:errorcluster)  [unwired: 9 in, 6 out]
                n98 = call "GFG_core.vi"("Variable Name in"="posY", "Variant in"=w321, "error in (no error)"=w326, "Action"=w334) -> ("error out"=w327:errorcluster)  [unwired: 9 in, 6 out]
                n99 = call "GFG_core.vi"("Variable Name in"="posZ", "Variant in"=w320, "error in (no error)"=w327, "Action"=w334) -> ("error out"=w328:errorcluster)  [unwired: 9 in, 6 out]
              }
              frame Disabled {
              }
            }
          }
          frame "posX", "posY", "posZ" {
            # "Invalidate Image when carriage moves"
            n100 = call "GetCurrentPosition.vi"("Error In"=w348) -> ("Error Out"=w346:errorcluster, "Z"=w351:dbl, "Y"=w350:dbl, "X"=w349:dbl)  [unwired: 7 in]
            n101 = call "Image Validity FGV.vi"("Image Validity FGV_Commands"=Image_Validity_FGV_Commands."Set validity status", "Error In"=w346, "Validity status IN"=FALSE) -> ("Error Out"=w344:errorcluster)  [unwired: 7 in, 1 out]
            n102 = call "GenerateDisplayData.vi"("Index"=w337, "Error In"=w344, "UI Controls Refnum"=w339, "2D Data IN"=w342) -> ("Error Out"=w343:errorcluster, "Plot Data OUT"=w341:cluster{dbl[], dbl[]}[])  [unwired: 4 in, 2 out]
          }
          frame "QUIT" {
            w379 = string[][] [] ("Formatted Table Data")
            w385 = 0.0 ("X")
            # "Reset the button in main UI"
            # "Clear table display"
            n103 = Unbundle By Name(w383) -> ("Big Table"=w377:refnum<vi>, "Notes Table"=w380:refnum<vi>, "Hide"=w372:refnum<vi>)
            n104 = Build Array(w377, w380) -> (w376:refnum<vi>[])
            n105 = call "FormatTableStyle.vi"("Format Command"=FormatTableStyle_Commands."Uncolour Row", "Error In"=w382, "Row Index"=w384, "Table reference Array"=w376) -> ("Error Out"=w381:errorcluster)  [unwired: 7 in]
            n106 = for {
              tunnel: w379 -> [w408]
              shift-right: [w407] -> w369
              shift-left: w381 -> [w411]
              tunnel: w376 -> [w406] mode=indexing
              n107 = property class="Tbl (strict)"(reference=w406, error in=w411, "Value"=w408) -> (reference out=w409:refnum<vi>, error out=w410:errorcluster)
              n108 = Close Reference(reference=w409, error in (no error)=w410) -> (error out=w407:errorcluster)
            }
            n109 = call "GFGfpRefGet.vi"("Variable Name in"="PositionSaveButton") -> ("output cluster"=w360:T21)  [unwired: 9 in, 1 out]
            n110 = Unbundle By Name(w360) -> ("BooleanRef"=w356:refnum<vi>)
            n111 = property class="Bool (strict)"(reference=w372, error in=w369, "Value"=T2 FALSE) -> (reference out=w370:refnum<vi>, error out=w371:errorcluster)
            n112 = control-ref of="This VI"() -> (w367:refnum<vi>)
            n113 = property class="Bool"(reference=w356, "Value"=FALSE) -> (reference out=w357:refnum<vi>, error out=w358:errorcluster)  [unwired: 1 in]
            n114 = Close Reference(reference=w370, error in (no error)=w371) -> (error out=w366:errorcluster)
            n115 = property class="VI"(reference=w367, error in=w366) -> (error out=w364:errorcluster, "FP.State"=w365:T12)  [unwired: 1 out]
            n116 = Close Reference(reference=w357, error in (no error)=w358) -> (error out=w352:errorcluster)
            n117 = case shown="\"Hidden\"" w365 {
              tunnel: [w388 w391 w396 w401 w404 w405] -> w363
              tunnel: w367 -> [_ w390 w395 w400 _ _]
              tunnel: w364 -> [w388 w389 w394 w399 w404 w405]
              frame "Invalid", Default {
              }
              frame "Standard" {
                n118 = invoke class="VI" method="FP.Close"(reference=w390, error in=w389) -> (reference out=w392:refnum<vi>, error out=w393:errorcluster)  [unwired: 1 in, 1 out]
                n119 = Close Reference(reference=w392, error in (no error)=w393) -> (error out=w391:errorcluster)
              }
              frame "Minimized" {
                n120 = invoke class="VI" method="FP.Close"(reference=w395, error in=w394) -> (reference out=w397:refnum<vi>, error out=w398:errorcluster)  [unwired: 1 in, 1 out]
                n121 = Close Reference(reference=w397, error in (no error)=w398) -> (error out=w396:errorcluster)
              }
              frame "Maximized" {
                n122 = invoke class="VI" method="FP.Close"(reference=w400, error in=w399) -> (reference out=w402:refnum<vi>, error out=w403:errorcluster)  [unwired: 1 in, 1 out]
                n123 = Close Reference(reference=w402, error in (no error)=w403) -> (error out=w401:errorcluster)
              }
              frame "Closed" {
              }
              frame "Hidden" {
              }
            }
            n124 = flat-sequence {
              tunnel: w363 -> [w386]
              tunnel: [w386] -> _
              tunnel: [TRUE] -> w355
              tunnel: [w386] -> w353
              frame #0 {
              }
            }
            n125 = Merge Errors(w353, w352) -> (w354:errorcluster)
          }
        }
      }
      event "Overlay": Value Change {
        # "Enable/Disable the Overlay cluster according to\nthe value"
        n126 = event-data() -> ("NewVal"=w417:bool)  [unwired: 1 in]
        n127 = Unbundle By Name(w416) -> ("Overlay Controls"=w415:refnum<vi>)
        n128 = case shown="False" w417 {
          tunnel: w415 -> [w429 w434]
          tunnel: w414 -> [w430 w435]
          tunnel: [w427 w432] -> w413
          frame True {
            n129 = Build Array(w429) -> (w428:refnum<vi>[])
            n130 = call "UI Control and Indicator properties.vi"("Enable Command"=UI_Control_and_Indicator_properties_Commands."Enable", "Error In"=w430, "Control Refnums"=w428) -> ("Error Out"=w427:errorcluster)  [unwired: 8 in]
          }
          frame False {
            n131 = Build Array(w434) -> (w433:refnum<vi>[])
            n132 = call "UI Control and Indicator properties.vi"("Enable Command"=UI_Control_and_Indicator_properties_Commands."Disable and Grey", "Error In"=w435, "Control Refnums"=w433) -> ("Error Out"=w432:errorcluster)  [unwired: 8 in]
          }
        }
      }
      event Value Change {
        # "Make sure the loop executes, to update the Image whenever there is a change in  any of the Overlay controls"
        n133 = event-data() -> ()  [unwired: 1 in, 1 out]
      }
      event "Hor_Cluster.Load List": Value Change {
        w470 = T11 {"CurrentImage"=refnum, "SavedImage"=refnum}  # Image Input Cluster
        # "Update table and plot display"
        n134 = event-data() -> ()  [unwired: 1 in, 1 out]
        n135 = Bundle By Name(cluster=w470, "CurrentImage"=w469, "SavedImage"=w468) -> (w467:T11)
        n136 = call "PositionSaveFGV.vi"("Image Cluster Input"=w467, "PositionSave Commands"=PositionSaveFGVCommands."LoadList", "Error In"=w475) -> ("Error Out"=w474:errorcluster, "SavedImage out"=w466:T7, "cancelled/failed"=w473:bool, "Position Data Out"=w476:string[][], "Path"=w465:path)  [unwired: 4 in]
        n137 = case shown="True" w473 {
          tunnel: w476 -> [w492 _]
          tunnel: w474 -> [w502 w517]
          tunnel: [w494 w517] -> w455
          tunnel: [w492 w516] -> w459
          tunnel: w450 -> [w486 _]
          tunnel: w472 -> [_ w516]
          tunnel: w471 -> [w482 w515]
          tunnel: [w481 w515] -> w458
          frame False {
            # "No of rows > 0?"
            # "Colour only if there\nare entries"
            # "Enable UI components and \nUpdate table and Graph"
            n138 = Unbundle By Name(w486) -> ("Set POI"=w483:refnum<vi>, "Set New Origin"=w507:refnum<vi>, "Delete Item"=w506:refnum<vi>, "Notes Table"=w496:refnum<vi>, "GO TO"=w505:refnum<vi>, "Big Table"=w484:refnum<vi>, "Table Up-End"=w501:refnum<vi>, "Table Up"=w500:refnum<vi>, "Table Down"=w499:refnum<vi>, "Table Down-End"=w498:refnum<vi>, "Copy Button"=w487:refnum<vi>)
            n139 = Build Array(w483, w507, w506, w496, w505, w484, w501, w500, w499, w498, w487) -> (w503:refnum<vi>[])
            n140 = Build Array(w496, w484) -> (w493:refnum<vi>[])
            n141 = call "UI Control and Indicator properties.vi"("Enable Command"=UI_Control_and_Indicator_properties_Commands."Enable", "Error In"=w502, "Control Refnums"=w503) -> ("Error Out"=w485:errorcluster)  [unwired: 8 in]
            n142 = Array Size(array=w492) -> (size(s)=w491:i32[])
            n143 = Index Array(array=w491, index=0) -> (element=w489:i32)
            n144 = Greater Than 0?(x=w489) -> (x > 0?=w488:bool)
            n145 = call "FormatTableStyle.vi"("Format Command"=FormatTableStyle_Commands."Uncolour Row", "Error In"=w485, "Row Index"=w482, "Table reference Array"=w493) -> ("Error Out"=w495:errorcluster)  [unwired: 7 in]
            n146 = case shown="False" w488 {
              tunnel: w495 -> [w509 w514]
              tunnel: [w509 w512] -> w494
              tunnel: w493 -> [_ w511]
              tunnel: [-1 ("Row") w510] -> w481
              frame False {
              }
              frame True {
                w510 = 0 ("Row")
                n147 = call "FormatTableStyle.vi"("Format Command"=FormatTableStyle_Commands."Colour Row", "Error In"=w514, "Row Index"=w510, "Table reference Array"=w511) -> ("Error Out"=w512:errorcluster)  [unwired: 7 in]
              }
            }
          }
          frame True {
            # "Action cancelled by user\n- Do nothing"
          }
        }
        n148 = call "GenerateDisplayData.vi"("Index"=w458, "Error In"=w455, "UI Controls Refnum"=w450, "2D Data IN"=w459) -> ("Error Out"=w451:errorcluster, "Notes"=w452:string[][], "Big Table"=w462:string[][], "Plot Data OUT"=w457:cluster{dbl[], dbl[]}[])  [unwired: 4 in]
        n149 = Unbundle By Name(w450) -> ("Big Table"=w456:refnum<vi>, "Notes Table"=w453:refnum<vi>)
        n150 = property class="Tbl (strict)"(reference=w456, error in=w451, "Value"=w462) -> (reference out=w463:refnum<vi>, error out=w464:errorcluster)
        n151 = Close Reference(reference=w463, error in (no error)=w464) -> (error out=w454:errorcluster)
        n152 = property class="Tbl (strict)"(reference=w453, error in=w454, "Value"=w452) -> (reference out=w460:refnum<vi>, error out=w461:errorcluster)
        n153 = Close Reference(reference=w460, error in (no error)=w461) -> (error out=w449:errorcluster)
      }
      event "Hor_Cluster.New List": Value Change {
        n154 = event-data() -> ()  [unwired: 1 in, 1 out]
        n155 = Bundle By Name(cluster=T11 {"CurrentImage"=refnum, "SavedImage"=refnum} ("Image Cluster Input"), "CurrentImage"=w529, "SavedImage"=w530) -> (w528:T11)
        n156 = call "PositionSaveFGV.vi"("Image Cluster Input"=w528, "PositionSave Commands"=PositionSaveFGVCommands."NewList", "Error In"=w535) -> ("Error Out"=w534:errorcluster, "SavedImage out"=w527:T7, "cancelled/failed"=w533:bool, "Position Data Out"=w536:string[][], "Path"=w525:path)  [unwired: 4 in]
        n157 = case shown="True" w533 {
          tunnel: w536 -> [w551 _]
          tunnel: w534 -> [w563 w574]
          tunnel: [w548 w574] -> w524
          tunnel: [w551 w573] -> w523
          tunnel: w519 -> [w542 _]
          tunnel: w532 -> [_ w573]
          tunnel: w531 -> [w556 w572]
          tunnel: [0 ("Row") w572] -> w520
          frame False {
            # "Enable UI components and \nUpdate table and Graph"
            n158 = Unbundle By Name(w542) -> ("Set New Origin"=w543:refnum<vi>, "Notes Table"=w544:refnum<vi>, "Big Table"=w555:refnum<vi>, "Table Up-End"=w562:refnum<vi>, "Table Up"=w561:refnum<vi>, "Table Down"=w560:refnum<vi>, "Table Down-End"=w559:refnum<vi>, "Copy Button"=w545:refnum<vi>)  [unwired: 1 out]
            n159 = Build Array(w544, w555) -> (w552:refnum<vi>[])
            n160 = Build Array(w543, w544, w555, w562, w561, w560, w559, w545) -> (w564:refnum<vi>[])
            n161 = call "UI Control and Indicator properties.vi"("Enable Command"=UI_Control_and_Indicator_properties_Commands."Enable", "Error In"=w563, "Control Refnums"=w564) -> ("Error Out"=w541:errorcluster)  [unwired: 8 in]
            n162 = call "FormatTableStyle.vi"("Format Command"=FormatTableStyle_Commands."Uncolour Row", "Error In"=w541, "Row Index"=w556, "Table reference Array"=w552) -> ("Error Out"=w554:errorcluster)  [unwired: 7 in]
            n163 = for {
              tunnel: string[][] [] ("Value") -> [w570]
              shift-right: [w567] -> w547
              shift-left: w554 -> [w571]
              tunnel: w552 -> [w566] mode=indexing
              n164 = property class="Tbl (strict)"(reference=w566, error in=w571, "Value"=w570) -> (reference out=w568:refnum<vi>, error out=w569:errorcluster)
              n165 = Close Reference(reference=w568, error in (no error)=w569) -> (error out=w567:errorcluster)
            }
            n166 = property class="Bool"(reference=w543, error in=w547, "Blinking"=TRUE) -> (reference out=w549:refnum<vi>, error out=w550:errorcluster)
            n167 = Close Reference(reference=w549, error in (no error)=w550) -> (error out=w548:errorcluster)
          }
          frame True {
            # "Action cancelled by user\n- Do nothing"
          }
        }
        n168 = call "GenerateDisplayData.vi"("Index"=w520, "Error In"=w524, "UI Controls Refnum"=w519, "2D Data IN"=w523) -> ("Error Out"=w521:errorcluster, "Plot Data OUT"=w522:cluster{dbl[], dbl[]}[])  [unwired: 4 in, 2 out]
      }
      event "Hor_Cluster.Set new Origin": Value Change {
        w596 = T11 {"CurrentImage"=refnum, "SavedImage"=refnum}  # Image Input Cluster
        # "Is there any data in the\nlist?"
        # "If the image is not up-to-date donot set POI!"
        n169 = event-data() -> ()  [unwired: 1 in, 1 out]
        n170 = Array Size(array=w584) -> (size(s)=w583:i32[])
        n171 = Bundle By Name(cluster=w596, "CurrentImage"=w594, "SavedImage"=w595) -> (w593:T11)
        n172 = call "Image Validity FGV.vi"("Image Validity FGV_Commands"=Image_Validity_FGV_Commands."Get Validity status", "Error In"=w588) -> ("Error Out"=w586:errorcluster, "Validity status OUT"=w585:bool)  [unwired: 8 in]
        n173 = Index Array(array=w583, index=0) -> (element=w581:i32)
        n174 = Greater Than 0?(x=w581) -> (x > 0?=w580:bool)
        n175 = case shown="False" w585 {
          tunnel: w604 -> [w608 w622]
          tunnel: w603 -> [w607 w621]
          tunnel: w591 -> [w606 w620]
          tunnel: w586 -> [w613 w618]
          tunnel: [w614 w633] -> w602
          tunnel: w579 -> [_ w632]
          tunnel: [w613 w631] -> w601
          tunnel: w584 -> [w614 w630]
          tunnel: w600 -> [w612 w628]
          tunnel: [w612 w627] -> w599
          tunnel: w598 -> [w609 w626]
          tunnel: [w609 w625] -> w597
          tunnel: w593 -> [w611 w624]
          tunnel: [w610 w623] -> w576
          tunnel: [w608 w622] -> w592
          tunnel: [w607 w621] -> w590
          tunnel: [w606 w620] -> w589
          tunnel: w580 -> [_ w619]
          tunnel: [w605 w617] -> w578
          tunnel: w577 -> [w605 w616]
          frame False {
            n176 = Unbundle By Name(w611) -> ("SavedImage"=w610:T7)
            n177 = call "Dialog_ImageNotUptodate_Error.vi"() -> ()  [unwired: 12 in]
          }
          frame True {
            w635 = T19 {"X"=0.0, "Y"=0.0, "Z"=0.0, "Base Path"=path ""}  # Position Data In
            # "Takes the current XYZ position and updates the table data on user confirmation"
            n178 = case shown="True" w619 {
              selector: w619 -> [w636 w639]
              tunnel: [TRUE ("T button?") w638] -> w629
              tunnel: [w636 w639] -> w615
              frame False {
              }
              frame True {
                n179 = call "Dialog_SetNewOrigin.vi"() -> ("OK?"=w638:bool)  [unwired: 11 in]
              }
            }
            n180 = Bundle By Name(cluster=w635, "X"=w622, "Y"=w621, "Z"=w620) -> (w634:T19)
            n181 = case shown="True" w629 {
              tunnel: w618 -> [w645 w686]
              tunnel: w634 -> [_ w685]
              tunnel: [w646 w684] -> w633
              tunnel: w632 -> [_ w649]
              tunnel: [w645 w654] -> w631
              tunnel: w630 -> [w646 _]
              tunnel: w628 -> [w644 w648]
              tunnel: [w644 w673] -> w627
              tunnel: w626 -> [w643 _]
              tunnel: [w643 w664] -> w625
              tunnel: w624 -> [w642 w663]
              tunnel: [w641 w662] -> w623
              tunnel: [w640 w651] -> w617
              tunnel: w616 -> [w640 _]
              tunnel: w615 -> [_ w650]
              frame False {
                n182 = Unbundle By Name(w642) -> ("SavedImage"=w641:T7)
              }
              frame True {
                w673 = 0 ("Row Index")
                # "If this is a new data file,\nenable the 'Go To' and 'Delete buttons'"
                n183 = call "PositionSaveFGV.vi"("Image Cluster Input"=w663, "PositionSave Commands"=PositionSaveFGVCommands."SetNewOrigin", "Error In"=w686, "Position Data In"=w685) -> ("Error Out"=w665:errorcluster, "SavedImage out"=w662:T7, "Position Data Out"=w684:string[][], "Path"=w651:path)  [unwired: 3 in, 1 out]
                n184 = Unbundle By Name(w649) -> ("Big Table"=w682:refnum<vi>, "Notes Table"=w669:refnum<vi>, "Set New Origin"=w660:refnum<vi>, "Set POI"=w656:refnum<vi>)
                n185 = case shown="False" w650 {
                  tunnel: w649 -> [w692 _]
                  frame False {
                    n186 = Unbundle By Name(w692) -> ("GO TO"=w690:refnum<vi>, "Delete Item"=w689:refnum<vi>)
                    n187 = Build Array(w690, w689) -> (w688:refnum<vi>[])
                    n188 = call "UI Control and Indicator properties.vi"("Enable Command"=UI_Control_and_Indicator_properties_Commands."Enable", "Control Refnums"=w688) -> ()  [unwired: 9 in, 1 out]
                  }
                  frame True {
                  }
                }
                n189 = call "GenerateDisplayData.vi"("Index"=0, "Error In"=w665, "UI Controls Refnum"=w649, "2D Data IN"=w684) -> ("Error Out"=w683:errorcluster, "Notes"=w666:string[][], "Big Table"=w667:string[][], "Plot Data OUT"=w664:cluster{dbl[], dbl[]}[])  [unwired: 4 in]
                n190 = property class="Tbl (strict)"(reference=w682, error in=w683, "Value"=w667) -> (reference out=w680:refnum<vi>, error out=w681:errorcluster)
                n191 = Build Array(w682, w669) -> (w675:refnum<vi>[])
                n192 = Build Array(w656) -> (w653:refnum<vi>[])
                n193 = Close Reference(reference=w680, error in (no error)=w681) -> (error out=w672:errorcluster)
                n194 = property class="Tbl (strict)"(reference=w669, error in=w672, "Value"=w666) -> (reference out=w670:refnum<vi>, error out=w671:errorcluster)
                n195 = Close Reference(reference=w670, error in (no error)=w671) -> (error out=w668:errorcluster)
                n196 = call "FormatTableStyle.vi"("Format Command"=FormatTableStyle_Commands."Uncolour Row", "Error In"=w668, "Row Index"=w648, "Table reference Array"=w675) -> ("Error Out"=w676:errorcluster)  [unwired: 7 in]
                n197 = call "FormatTableStyle.vi"("Format Command"=FormatTableStyle_Commands."Colour Row", "Error In"=w676, "Row Index"=w673, "Table reference Array"=w675) -> ("Error Out"=w674:errorcluster)  [unwired: 7 in]
                n198 = call "FormatTableStyle.vi"("Format Command"=FormatTableStyle_Commands."UpdateVisibleRows", "Error In"=w674, "Row Index"=w673, "Table reference Array"=w675) -> ("Error Out"=w661:errorcluster)  [unwired: 7 in]
                n199 = property class="Bool"(reference=w660, error in=w661, "Blinking"=FALSE) -> (reference out=w657:refnum<vi>, error out=w658:errorcluster)
                n200 = Close Reference(reference=w657, error in (no error)=w658) -> (error out=w655:errorcluster)
                n201 = call "UI Control and Indicator properties.vi"("Enable Command"=UI_Control_and_Indicator_properties_Commands."Enable", "Error In"=w655, "Control Refnums"=w653) -> ("Error Out"=w654:errorcluster)  [unwired: 8 in]
              }
            }
          }
        }
      }
      event "Copy Button": Value Change {
        w699 = T11 {"CurrentImage"=refnum, "SavedImage"=refnum}  # Image Input Cluster
        # "Makes a copy of the csv file to user specified destination. For implementation details check the PositionSaveFGV."
        n202 = event-data() -> ()  [unwired: 1 in, 1 out]
        n203 = Bundle By Name(cluster=w699, "CurrentImage"=w698, "SavedImage"=w697) -> (w696:T11)
        n204 = call "PositionSaveFGV.vi"("Image Cluster Input"=w696, "PositionSave Commands"=PositionSaveFGVCommands."CopyList", "Error In"=w710) -> ("Error Out"=w709:errorcluster, "SavedImage out"=w695:T7, "cancelled/failed"=w704:bool, "Position Data Out"=w711:string[][], "Path"=w694:path)  [unwired: 4 in]
        n205 = case shown="False" w704 {
          tunnel: w711 -> [w727 _]
          tunnel: w709 -> [w743 w759]
          tunnel: [w730 w759] -> w708
          tunnel: [w727 w758] -> w707
          tunnel: [w722 w760] -> w706
          tunnel: w705 -> [_ w760]
          tunnel: w703 -> [w717 _]
          tunnel: w702 -> [_ w758]
          tunnel: w701 -> [w716 w757]
          tunnel: [w728 w757] -> w700
          frame False {
            w728 = 0 ("Row")
            # "No of rows > 0?"
            # "Colour only if there\nare entries"
            # "Enable UI components and \nUpdate table and Graph"
            n206 = Unbundle By Name(w717) -> ("Set POI"=w719:refnum<vi>, "Set New Origin"=w750:refnum<vi>, "Delete Item"=w749:refnum<vi>, "Notes Table"=w734:refnum<vi>, "GO TO"=w748:refnum<vi>, "Big Table"=w733:refnum<vi>, "Table Up-End"=w742:refnum<vi>, "Table Up"=w741:refnum<vi>, "Table Down"=w740:refnum<vi>, "Table Down-End"=w739:refnum<vi>, "Copy Button"=w718:refnum<vi>)
            n207 = Build Array(w719, w750, w749, w734, w748, w733, w742, w741, w740, w739, w718) -> (w746:refnum<vi>[])
            n208 = call "UI Control and Indicator properties.vi"("Enable Command"=UI_Control_and_Indicator_properties_Commands."Enable", "Error In"=w743, "Control Refnums"=w746) -> ("Error Out"=w745:errorcluster)  [unwired: 8 in]
            n209 = call "GenerateDisplayData.vi"("Index"=w716, "Error In"=w745, "UI Controls Refnum"=w717, "2D Data IN"=w727) -> ("Error Out"=w744:errorcluster, "Notes"=w720:string[][], "Big Table"=w721:string[][], "Plot Data OUT"=w722:cluster{dbl[], dbl[]}[])  [unwired: 4 in]
            n210 = property on="Notes_Table" class="Tbl (strict)"(error in=w744, "Value"=w720) -> (error out=w738:errorcluster)  [unwired: 1 in, 1 out]
            n211 = Build Array(w734, w733) -> (w729:refnum<vi>[])
            n212 = property class="Tbl (strict)"(reference=w733, error in=w738, "Value"=w721) -> (reference out=w736:refnum<vi>, error out=w737:errorcluster)
            n213 = Array Size(array=w727) -> (size(s)=w726:i32[])
            n214 = Close Reference(reference=w736, error in (no error)=w737) -> (error out=w732:errorcluster)
            n215 = Index Array(array=w726, index=0) -> (element=w724:i32)
            n216 = Greater Than 0?(x=w724) -> (x > 0?=w723:bool)
            n217 = call "FormatTableStyle.vi"("Format Command"=FormatTableStyle_Commands."Uncolour Row", "Error In"=w732, "Row Index"=w716, "Table reference Array"=w729) -> ("Error Out"=w731:errorcluster)  [unwired: 7 in]
            n218 = case shown="True" w723 {
              tunnel: w731 -> [w751 w756]
              tunnel: [w751 w754] -> w730
              tunnel: w729 -> [_ w753]
              tunnel: w728 -> [_ w752]
              frame False {
              }
              frame True {
                n219 = call "FormatTableStyle.vi"("Format Command"=FormatTableStyle_Commands."Colour Row", "Error In"=w756, "Row Index"=w752, "Table reference Array"=w753) -> ("Error Out"=w754:errorcluster)  [unwired: 7 in]
              }
            }
          }
          frame True {
            # "Action cancelled by user\n- Do nothing"
          }
        }
      }
      event "Vert_Cluster.SET POI": Value Change {
        w783 = T11 {"CurrentImage"=refnum, "SavedImage"=refnum}  # Image Input Cluster
        # "Update plot and table"
        # "If the image is not up-to-date\ndonot set POI!"
        n220 = event-data() -> ()  [unwired: 1 in, 1 out]
        n221 = call "Image Validity FGV.vi"("Image Validity FGV_Commands"=Image_Validity_FGV_Commands."Get Validity status", "Error In"=w778) -> ("Error Out"=w777:errorcluster, "Validity status OUT"=w775:bool)  [unwired: 8 in]
        n222 = Bundle By Name(cluster=w783, "CurrentImage"=w782, "SavedImage"=w781) -> (w780:T11)
        n223 = case shown="False" w775 {
          tunnel: w777 -> [w791 w809]
          tunnel: w763 -> [_ w797]
          tunnel: w785 -> [w792 w808]
          tunnel: [w790 w807] -> w765
          tunnel: [w791 w806] -> w768
          tunnel: [w792 w805] -> w764
          tunnel: [w793 w804] -> w784
          tunnel: w780 -> [w794 w803]
          tunnel: w779 -> [w790 w795]
          tunnel: [w789 w802] -> w774
          tunnel: w773 -> [w789 w796]
          frame False {
            n224 = Unbundle By Name(w794) -> ("SavedImage"=w793:T7)
            n225 = call "Dialog_ImageNotUptodate_Error.vi"() -> ()  [unwired: 12 in]
          }
          frame True {
            # "Are there any saved\ndata points?"
            n226 = Array Size(array=w795) -> (size(s)=w801:i32[])
            n227 = Index Array(array=w801, index=0) -> (element=w799:i32)
            n228 = Greater Than 0?(x=w799) -> (x > 0?=w798:bool)
            n229 = case shown="False" w798 {
              tunnel: w809 -> [w813 w840]
              tunnel: w797 -> [_ w818]
              tunnel: w808 -> [w812 w817]
              tunnel: [w810 w830] -> w807
              tunnel: [w813 w826] -> w806
              tunnel: [w812 w825] -> w805
              tunnel: [w814 w824] -> w804
              tunnel: w803 -> [w815 w823]
              tunnel: [w811 w819] -> w802
              tunnel: w796 -> [w811 _]
              tunnel: w795 -> [w810 _]
              frame False {
                n230 = Unbundle By Name(w815) -> ("SavedImage"=w814:T7)
                n231 = call "Dialog_NoOrigin_Error.vi"() -> ()  [unwired: 12 in]
              }
              frame True {
                # "If there is atleast one row, add changes to the UI and update index acordingly"
                n232 = call "GetCurrentPosition.vi"("Error In"=w840) -> ("Error Out"=w834:errorcluster, "Z"=w835:dbl, "Y"=w836:dbl, "X"=w837:dbl)  [unwired: 7 in]
                n233 = Unbundle By Name(w818) -> ("Big Table"=w832:refnum<vi>, "Notes Table"=w831:refnum<vi>, "Set New Origin"=w820:refnum<vi>)
                n234 = Bundle By Name(cluster=T19 {"X"=0.0, "Y"=0.0, "Z"=0.0, "Base Path"=path ""} ("Position Data In"), "X"=w837, "Y"=w836, "Z"=w835) -> (w833:T19)
                n235 = call "PositionSaveFGV.vi"("Image Cluster Input"=w823, "PositionSave Commands"=PositionSaveFGVCommands."SetPosition", "Error In"=w834, "Position Data In"=w833) -> ("Error Out"=w816:errorcluster, "SavedImage out"=w824:T7, "Position Data Out"=w830:string[][], "Path"=w819:path)  [unwired: 3 in, 1 out]
                n236 = Build Array(w832, w831) -> (w827:refnum<vi>[])
                n237 = Array Size(array=w830) -> (size(s)=w829:i32[])
                n238 = Index Array(array=w829, index=0) -> (element=w822:i32)
                n239 = Greater Than 0?(x=w822) -> (x > 0?=w821:bool)
                n240 = case shown="True" w821 {
                  tunnel: w817 -> [_ w857]
                  tunnel: w816 -> [w842 w855]
                  tunnel: w827 -> [_ w851]
                  tunnel: [w842 w848] -> w826
                  tunnel: [w841 w850] -> w825
                  tunnel: w822 -> [w841 w849]
                  tunnel: w820 -> [_ w845]
                  frame False {
                  }
                  frame True {
                    n241 = Decrement(x=w849) -> (x-1=w850:i32)
                    n242 = call "FormatTableStyle.vi"("Format Command"=FormatTableStyle_Commands."Uncolour Row", "Error In"=w855, "Row Index"=w857, "Table reference Array"=w851) -> ("Error Out"=w852:errorcluster)  [unwired: 7 in]
                    n243 = call "FormatTableStyle.vi"("Format Command"=FormatTableStyle_Commands."Colour Row", "Error In"=w852, "Row Index"=w850, "Table reference Array"=w851) -> ("Error Out"=w853:errorcluster)  [unwired: 7 in]
                    n244 = call "FormatTableStyle.vi"("Format Command"=FormatTableStyle_Commands."UpdateVisibleRows", "Error In"=w853, "Row Index"=w850, "Table reference Array"=w851) -> ("Error Out"=w844:errorcluster)  [unwired: 7 in]
                    n245 = property class="Bool"(reference=w845, error in=w844, "Blinking"=FALSE) -> (reference out=w846:refnum<vi>, error out=w847:errorcluster)
                    n246 = Close Reference(reference=w846, error in (no error)=w847) -> (error out=w848:errorcluster)
                  }
                }
              }
            }
          }
        }
        n247 = Unbundle By Name(w763) -> ("Big Table"=w766:refnum<vi>)
        n248 = call "GenerateDisplayData.vi"("Index"=w764, "Error In"=w768, "UI Controls Refnum"=w763, "2D Data IN"=w765) -> ("Error Out"=w772:errorcluster, "Big Table"=w769:string[][], "Plot Data OUT"=w762:cluster{dbl[], dbl[]}[])  [unwired: 4 in, 1 out]
        n249 = property class="Tbl (strict)"(reference=w766, error in=w772, "Value"=w769) -> (reference out=w770:refnum<vi>, error out=w771:errorcluster)
        n250 = Close Reference(reference=w770, error in (no error)=w771) -> (error out=w767:errorcluster)
      }
      event "Vert_Cluster.Delete item": Value Change {
        # "Is there any saved positions?\n(Other than origin)"
        n251 = event-data() -> ()  [unwired: 1 in, 1 out]
        n252 = Greater Than 0?(x=w868) -> (x > 0?=w862:bool)
        n253 = Bundle By Name(cluster=T11 {"CurrentImage"=refnum, "SavedImage"=refnum} ("Image Input Cluster"), "SavedImage"=w866, "CurrentImage"=w865) -> (w864:T11)
        n254 = case shown="False" w862 {
          selector: w862 -> [w880 _]
          tunnel: w868 -> [w885 w900]
          tunnel: w876 -> [w886 w901]
          tunnel: w875 -> [w887 w899]
          tunnel: [w886 w898] -> w874
          tunnel: [w885 w897] -> w873
          tunnel: w872 -> [_ w896]
          tunnel: [w887 w895] -> w871
          tunnel: [w884 w894] -> w870
          tunnel: w869 -> [w884 w893]
          tunnel: w864 -> [w883 w892]
          tunnel: [w882 w891] -> w863
          tunnel: [w881 w890] -> w861
          tunnel: w860 -> [w881 w889]
          frame False {
            n255 = Unbundle By Name(w883) -> ("SavedImage"=w882:T7)
            n256 = case shown="False" w880 {
              frame False {
                n257 = call "Dialog_DeleteOrigin_Error.vi"() -> ()  [unwired: 12 in]
              }
              frame True {
              }
            }
          }
          frame True {
            n258 = call "Dialog_DeleteConfirm.vi"() -> ("OK?"=w888:bool)  [unwired: 11 in]
            n259 = case shown="True" w888 {
              tunnel: w901 -> [w908 w923]
              tunnel: w900 -> [w907 w911]
              tunnel: w899 -> [w906 w922]
              tunnel: [w908 w920] -> w898
              tunnel: [w907 w910] -> w897
              tunnel: w896 -> [_ w921]
              tunnel: [w906 w919] -> w895
              tunnel: [w905 w917] -> w894
              tunnel: w893 -> [w905 w916]
              tunnel: w892 -> [w904 w914]
              tunnel: [w903 w913] -> w891
              tunnel: [w902 w909] -> w890
              tunnel: w889 -> [w902 _]
              frame False {
                n260 = Unbundle By Name(w904) -> ("SavedImage"=w903:T7)
              }
              frame True {
                n261 = call "PositionSaveFGV.vi"("Image Cluster Input"=w914, "PositionSave Commands"=PositionSaveFGVCommands."DeleteSelected", "Error In"=w922, "CompleteTableString"=w923, "Table Index"=w911) -> ("Error Out"=w918:errorcluster, "SavedImage out"=w913:T7, "cancelled/failed"=w915:bool, "Position Data Out"=w920:string[][], "Path"=w909:path)  [unwired: 2 in]
                n262 = Decrement(x=w911) -> (x-1=w912:i32)
                n263 = case shown="False" w915 {
                  tunnel: w921 -> [w926 _]
                  tunnel: w920 -> [w939 _]
                  tunnel: [w932 w950] -> w919
                  tunnel: w918 -> [w929 w950]
                  tunnel: [w928 w951] -> w917
                  tunnel: w916 -> [_ w951]
                  tunnel: w912 -> [w925 _]
                  tunnel: w911 -> [w927 w949]
                  tunnel: [w925 w949] -> w910
                  frame False {
                    n264 = Unbundle By Name(w926) -> ("Big Table"=w938:refnum<vi>, "Notes Table"=w936:refnum<vi>)
                    n265 = call "GenerateDisplayData.vi"("Index"=w925, "Error In"=w929, "UI Controls Refnum"=w926, "2D Data IN"=w939) -> ("Error Out"=w937:errorcluster, "Notes"=w931:string[][], "Big Table"=w930:string[][], "Plot Data OUT"=w928:cluster{dbl[], dbl[]}[])  [unwired: 4 in]
                    n266 = property class="Tbl (strict)"(reference=w938, error in=w937, "Value"=w930) -> (reference out=w943:refnum<vi>, error out=w942:errorcluster)
                    n267 = Close Reference(reference=w943, error in (no error)=w942) -> (error out=w941:errorcluster)
                    n268 = property class="Tbl (strict)"(reference=w936, error in=w941, "Value"=w931) -> (reference out=w944:refnum<vi>, error out=w945:errorcluster)
                    n269 = Build Array(w938, w936) -> (w933:refnum<vi>[])
                    n270 = Close Reference(reference=w944, error in (no error)=w945) -> (error out=w940:errorcluster)
                    n271 = call "FormatTableStyle.vi"("Format Command"=FormatTableStyle_Commands."Uncolour Row", "Error In"=w940, "Row Index"=w927, "Table reference Array"=w933) -> ("Error Out"=w947:errorcluster)  [unwired: 7 in]
                    n272 = call "FormatTableStyle.vi"("Format Command"=FormatTableStyle_Commands."Colour Row", "Error In"=w947, "Row Index"=w925, "Table reference Array"=w933) -> ("Error Out"=w935:errorcluster)  [unwired: 7 in]
                    n273 = call "FormatTableStyle.vi"("Format Command"=FormatTableStyle_Commands."UpdateVisibleRows", "Error In"=w935, "Row Index"=w925, "Table reference Array"=w933) -> ("Error Out"=w932:errorcluster)  [unwired: 7 in]
                  }
                  frame True {
                  }
                }
              }
            }
          }
        }
      }
      event "Big_Table": Mouse Up {
        w964 = T11 {"CurrentImage"=refnum, "SavedImage"=refnum}  # Image Input Cluster
        # "Did user click on a row within the data range?"
        n274 = event-data() -> ()  [unwired: 1 in, 1 out]
        n275 = Unbundle By Name(w953) -> ("Big Table"=w970:refnum<vi>, "Notes Table"=w971:refnum<vi>)
        n276 = Array Size(array=w957) -> (size(s)=w968:i32[])
        n277 = Index Array(array=w968, index=0) -> (element=w967:i32)
        n278 = Bundle By Name(cluster=w964, "SavedImage"=w963, "CurrentImage"=w962) -> (w961:T11)
        n279 = Decrement(x=w967) -> (x-1=w976:i32)
        n280 = property class="Tbl (strict)"(reference=w970, error in=w978) -> (reference out=w973:refnum<vi>, error out=w974:errorcluster, "Selection Start"=w977:T22)
        n281 = Build Array(w970, w971) -> (w969:refnum<vi>[])
        n282 = Close Reference(reference=w973, error in (no error)=w974) -> (error out=w972:errorcluster)
        n283 = Unbundle By Name(w977) -> ("Row"=w966:i32)
        n284 = Less Or Equal?(x=w966, y=w976) -> (x <= y?=w965:bool)
        n285 = case shown="True" w965 {
          tunnel: w966 -> [_ w988]
          tunnel: w975 -> [w986 w999]
          tunnel: [w986 w988] -> w955
          tunnel: w972 -> [w985 w1002]
          tunnel: w969 -> [_ w1001]
          tunnel: [w985 w991] -> w958
          tunnel: [w983 w990] -> w960
          tunnel: w957 -> [_ w989]
          tunnel: w961 -> [w984 w987]
          frame False {
            n286 = Unbundle By Name(w984) -> ("SavedImage"=w983:T7)
          }
          frame True {
            # "Update index, and highlight\ntable"
            n287 = call "FormatTableStyle.vi"("Format Command"=FormatTableStyle_Commands."Uncolour Row", "Error In"=w1002, "Row Index"=w999, "Table reference Array"=w1001) -> ("Error Out"=w1000:errorcluster)  [unwired: 7 in]
            n288 = call "FormatTableStyle.vi"("Format Command"=FormatTableStyle_Commands."Colour Row", "Error In"=w1000, "Row Index"=w988, "Table reference Array"=w1001) -> ("Error Out"=w992:errorcluster)  [unwired: 7 in]
            n289 = Index Array(array=w989, index (row)=w988, index (col)=8 ("disabled index (col)")) -> (element=w995:string)
            n290 = String To Path(string=w995) -> (path=w993:path)
            n291 = call "ImageIO.vi"("Pos_ImageIO_commands"=ImageIO_commands."ReadImage", "Error In"=w992, "Image File Path"=w993, "ImageCluster IN"=w987) -> ("Error Out"=w991:errorcluster, "Saved Image OUT"=w990:T7)  [unwired: 5 in, 1 out]
          }
        }
        n292 = call "GenerateDisplayData.vi"("Index"=w955, "Error In"=w958, "UI Controls Refnum"=w953, "2D Data IN"=w957) -> ("Error Out"=w954:errorcluster, "Plot Data OUT"=w956:cluster{dbl[], dbl[]}[])  [unwired: 4 in, 2 out]
      }
      event "Notes_Table": Mouse Up {
        w1016 = T11 {"CurrentImage"=refnum, "SavedImage"=refnum}  # Image Input Cluster
        # "Did user click on a row within the data range?"
        n293 = event-data() -> ()  [unwired: 1 in, 1 out]
        n294 = Unbundle By Name(w1004) -> ("Big Table"=w1022:refnum<vi>, "Notes Table"=w1010:refnum<vi>)
        n295 = Array Size(array=w1006) -> (size(s)=w1020:i32[])
        n296 = Index Array(array=w1020, index=0) -> (element=w1019:i32)
        n297 = Bundle By Name(cluster=w1016, "SavedImage"=w1015, "CurrentImage"=w1014) -> (w1013:T11)
        n298 = Decrement(x=w1019) -> (x-1=w1027:i32)
        n299 = property class="Tbl (strict)"(reference=w1010, error in=w1029) -> (reference out=w1024:refnum<vi>, error out=w1025:errorcluster, "Selection Start"=w1028:T22)
        n300 = Build Array(w1022, w1010) -> (w1021:refnum<vi>[])
        n301 = Close Reference(reference=w1024, error in (no error)=w1025) -> (error out=w1023:errorcluster)
        n302 = Unbundle By Name(w1028) -> ("Row"=w1018:i32)
        n303 = Less Or Equal?(x=w1018, y=w1027) -> (x <= y?=w1017:bool)
        n304 = case shown="False" w1017 {
          tunnel: w1018 -> [_ w1039]
          tunnel: w1026 -> [w1037 w1050]
          tunnel: [w1037 w1039] -> w1009
          tunnel: w1023 -> [w1036 w1053]
          tunnel: w1021 -> [_ w1052]
          tunnel: [w1036 w1042] -> w1008
          tunnel: [w1034 w1041] -> w1012
          tunnel: w1006 -> [_ w1040]
          tunnel: w1013 -> [w1035 w1038]
          frame False {
            n305 = Unbundle By Name(w1035) -> ("SavedImage"=w1034:T7)
          }
          frame True {
            # "Update index, and highlight\ntable"
            n306 = call "FormatTableStyle.vi"("Format Command"=FormatTableStyle_Commands."Uncolour Row", "Error In"=w1053, "Row Index"=w1050, "Table reference Array"=w1052) -> ("Error Out"=w1051:errorcluster)  [unwired: 7 in]
            n307 = call "FormatTableStyle.vi"("Format Command"=FormatTableStyle_Commands."Colour Row", "Error In"=w1051, "Row Index"=w1039, "Table reference Array"=w1052) -> ("Error Out"=w1043:errorcluster)  [unwired: 7 in]
            n308 = Index Array(array=w1040, index (row)=w1039, index (col)=8 ("disabled index (col)")) -> (element=w1046:string)
            n309 = String To Path(string=w1046) -> (path=w1044:path)
            n310 = call "ImageIO.vi"("Pos_ImageIO_commands"=ImageIO_commands."ReadImage", "Error In"=w1043, "Image File Path"=w1044, "ImageCluster IN"=w1038) -> ("Error Out"=w1042:errorcluster, "Saved Image OUT"=w1041:T7)  [unwired: 5 in, 1 out]
          }
        }
        n311 = call "GenerateDisplayData.vi"("Index"=w1009, "Error In"=w1008, "UI Controls Refnum"=w1004, "2D Data IN"=w1006) -> ("Error Out"=w1007:errorcluster, "Plot Data OUT"=w1005:cluster{dbl[], dbl[]}[])  [unwired: 4 in, 2 out]
      }
      event "Big_Table": Value Change {
        # "Dont allow user to manually change the vallues in the 'BIG Table'; roll back changes if \nany attempts are made.\nThis is done instead of disabling to alow greater user interactivity with teh table through\nselection (allowing user to click on columns anywhere in the table and taking appropriate action)"
        n312 = event-data() -> ("OldVal"=w1062:string[][])  [unwired: 1 in]
        n313 = Unbundle By Name(w1065) -> ("Big Table"=w1064:refnum<vi>)
        n314 = property class="Tbl (strict)"(reference=w1064, error in=w1063, "Value"=w1062) -> (reference out=w1060:refnum<vi>, error out=w1061:errorcluster)
        n315 = Close Reference(reference=w1060, error in (no error)=w1061) -> (error out=w1059:errorcluster)
        n316 = call "Dialog_CannotEdit_Error.vi"() -> ()  [unwired: 12 in]
      }
      event "Notes_Table": Value Change {
        # "Is selection within range?"
        # "are there any rows?"
        n317 = event-data() -> ("NewVal"=w1087:string[][])  [unwired: 1 in]
        n318 = Array Size(array=w1085) -> (size(s)=w1084:i32[])
        n319 = Index Array(array=w1084, index=0) -> (element=w1077:i32)
        n320 = Increment(x=w1072) -> (x+1=w1078:i32)
        n321 = Less Or Equal?(x=w1078, y=w1077) -> (x <= y?=w1075:bool)
        n322 = Greater?(x=w1077, y=0) -> (0:w1076:bool)
        n323 = And(x=w1075, y=w1076) -> (x .and. y?=w1074:bool)
        n324 = case shown="True" w1074 {
          tunnel: w1081 -> [w1100 w1118]
          tunnel: [w1101 w1107] -> w1088
          tunnel: w1085 -> [w1101 w1117]
          tunnel: w1087 -> [_ w1116]
          tunnel: [w1097 w1109] -> w1086
          tunnel: w1073 -> [w1095 w1110]
          tunnel: w1072 -> [_ w1108]
          frame False {
            # "Discard changes"
            n325 = Unbundle By Name(w1095) -> ("Notes Table"=w1094:refnum<vi>)
            n326 = property class="Tbl (strict)"(reference=w1094, error in=w1100, "Value"=string[][] []) -> (reference out=w1096:refnum<vi>, error out=w1098:errorcluster)
            n327 = Close Reference(reference=w1096, error in (no error)=w1098) -> (error out=w1097:errorcluster)
          }
          frame True {
            # "Update Table UI"
            # "modify notes field"
            # "get new notes"
            # "Write notes to File.\nIf failed, donot update"
            n328 = Index Array(array=w1116, index (col)=0 ("disabled index (col)")) -> (element=w1113:string[])  [unwired: 1 in]
            n329 = Replace Array Subset(array=w1117, new element=w1113, index (col)=7 ("disabled index (col)")) -> (w1112:string[][])  [unwired: 1 in]
            n330 = call "PositionSaveFGV.vi"("PositionSave Commands"=PositionSaveFGVCommands."UpdateEntireTable", "Error In"=w1118, "CompleteTableString"=w1112) -> ("Error Out"=w1111:errorcluster, "Position Data Out"=w1107:string[][])  [unwired: 4 in, 3 out]
            n331 = call "GenerateDisplayData.vi"("Index"=w1108, "Error In"=w1111, "UI Controls Refnum"=w1110, "2D Data IN"=w1107) -> ("Error Out"=w1106:errorcluster, "Notes"=w1105:string[][])  [unwired: 4 in, 2 out]
            n332 = Unbundle By Name(w1110) -> ("Notes Table"=w1104:refnum<vi>)
            n333 = property class="Tbl (strict)"(reference=w1104, error in=w1106, "Value"=w1105) -> (reference out=w1102:refnum<vi>, error out=w1103:errorcluster)
            n334 = Close Reference(reference=w1102, error in (no error)=w1103) -> (error out=w1109:errorcluster)
          }
        }
      }
      event "Table Navigation Cluster.Table Index Down": Value Change {
        # "No of rows"
        n335 = event-data() -> ()  [unwired: 1 in, 1 out]
        n336 = Unbundle By Name(w1122) -> ("Big Table"=w1141:refnum<vi>, "Notes Table"=w1140:refnum<vi>)
        n337 = Array Size(array=w1124) -> (size(s)=w1137:i32[])
        n338 = Bundle By Name(cluster=T11 {"CurrentImage"=refnum, "SavedImage"=refnum} ("Image Input Cluster"), "SavedImage"=w1131, "CurrentImage"=w1130) -> (w1129:T11)
        n339 = Index Array(array=w1137, index=0) -> (element=w1134:i32)
        n340 = Build Array(w1141, w1140) -> (w1139:refnum<vi>[])
        n341 = Decrement(x=w1134) -> (x-1=w1133:i32)
        n342 = Less?(x=w1135, y=w1133) -> (x < y?=w1142:bool)
        n343 = case shown="True" w1142 {
          tunnel: w1135 -> [w1149 w1167]
          tunnel: [w1149 w1158] -> w1126
          tunnel: w1139 -> [_ w1160]
          tunnel: w1138 -> [w1148 w1166]
          tunnel: [w1148 w1151] -> w1125
          tunnel: w1129 -> [w1147 w1153]
          tunnel: w1124 -> [_ w1159]
          tunnel: [w1146 w1150] -> w1128
          frame False {
            n344 = Unbundle By Name(w1147) -> ("SavedImage"=w1146:T7)
          }
          frame True {
            n345 = call "FormatTableStyle.vi"("Format Command"=FormatTableStyle_Commands."Uncolour Row", "Error In"=w1166, "Row Index"=w1167, "Table reference Array"=w1160) -> ("Error Out"=w1165:errorcluster)  [unwired: 7 in]
            n346 = Increment(x=w1167) -> (x+1=w1158:i32)
            n347 = call "FormatTableStyle.vi"("Format Command"=FormatTableStyle_Commands."Colour Row", "Error In"=w1165, "Row Index"=w1158, "Table reference Array"=w1160) -> ("Error Out"=w1161:errorcluster)  [unwired: 7 in]
            n348 = call "FormatTableStyle.vi"("Format Command"=FormatTableStyle_Commands."UpdateVisibleRows", "Error In"=w1161, "Row Index"=w1158, "Table reference Array"=w1160) -> ("Error Out"=w1152:errorcluster)  [unwired: 7 in]
            n349 = Index Array(array=w1159, index (row)=w1158, index (col)=8 ("disabled index (col)")) -> (element=w1156:string)
            n350 = String To Path(string=w1156) -> (path=w1154:path)
            n351 = call "ImageIO.vi"("Pos_ImageIO_commands"=ImageIO_commands."ReadImage", "Error In"=w1152, "Image File Path"=w1154, "ImageCluster IN"=w1153) -> ("Error Out"=w1151:errorcluster, "Saved Image OUT"=w1150:T7)  [unwired: 5 in, 1 out]
          }
        }
        n352 = call "GenerateDisplayData.vi"("Index"=w1126, "Error In"=w1125, "UI Controls Refnum"=w1122, "2D Data IN"=w1124) -> ("Error Out"=w1123:errorcluster, "Plot Data OUT"=w1121:cluster{dbl[], dbl[]}[])  [unwired: 4 in, 2 out]
      }
      event "Table Navigation Cluster.Table Index Down-End": Value Change {
        # "No of rows > 1?"
        n353 = event-data() -> ()  [unwired: 1 in, 1 out]
        n354 = Unbundle By Name(w1170) -> ("Big Table"=w1190:refnum<vi>, "Notes Table"=w1189:refnum<vi>)
        n355 = Bundle By Name(cluster=T11 {"CurrentImage"=refnum, "SavedImage"=refnum} ("Image Input Cluster"), "SavedImage"=w1179, "CurrentImage"=w1178) -> (w1177:T11)
        n356 = Array Size(array=w1171) -> (size(s)=w1188:i32[])
        n357 = Index Array(array=w1188, index=0) -> (element=w1182:i32)
        n358 = Build Array(w1190, w1189) -> (w1184:refnum<vi>[])
        n359 = Greater?(x=w1182, y=1) -> (0:w1183:bool)
        n360 = case shown="True" w1183 {
          tunnel: w1182 -> [w1196 w1216]
          tunnel: w1186 -> [w1197 w1212]
          tunnel: w1185 -> [_ w1211]
          tunnel: w1184 -> [_ w1210]
          tunnel: [w1197 w1199] -> w1174
          tunnel: [w1196 w1202] -> w1172
          tunnel: w1171 -> [_ w1203]
          tunnel: w1177 -> [w1195 w1200]
          tunnel: [w1194 w1198] -> w1176
          frame False {
            n361 = Unbundle By Name(w1195) -> ("SavedImage"=w1194:T7)
          }
          frame True {
            n362 = call "FormatTableStyle.vi"("Format Command"=FormatTableStyle_Commands."Uncolour Row", "Error In"=w1212, "Row Index"=w1211, "Table reference Array"=w1210) -> ("Error Out"=w1213:errorcluster)  [unwired: 7 in]
            n363 = Decrement(x=w1216) -> (x-1=w1202:i32)
            n364 = call "FormatTableStyle.vi"("Format Command"=FormatTableStyle_Commands."Colour Row", "Error In"=w1213, "Row Index"=w1202, "Table reference Array"=w1210) -> ("Error Out"=w1209:errorcluster)  [unwired: 7 in]
            n365 = call "FormatTableStyle.vi"("Format Command"=FormatTableStyle_Commands."UpdateVisibleRows", "Error In"=w1209, "Row Index"=w1202, "Table reference Array"=w1210) -> ("Error Out"=w1201:errorcluster)  [unwired: 7 in]
            n366 = Index Array(array=w1203, index (row)=w1202, index (col)=8 ("disabled index (col)")) -> (element=w1206:string)
            n367 = String To Path(string=w1206) -> (path=w1204:path)
            n368 = call "ImageIO.vi"("Pos_ImageIO_commands"=ImageIO_commands."ReadImage", "Error In"=w1201, "Image File Path"=w1204, "ImageCluster IN"=w1200) -> ("Error Out"=w1199:errorcluster, "Saved Image OUT"=w1198:T7)  [unwired: 5 in, 1 out]
          }
        }
        n369 = call "GenerateDisplayData.vi"("Index"=w1172, "Error In"=w1174, "UI Controls Refnum"=w1170, "2D Data IN"=w1171) -> ("Error Out"=w1173:errorcluster, "Plot Data OUT"=w1169:cluster{dbl[], dbl[]}[])  [unwired: 4 in, 2 out]
      }
      event "Table Navigation Cluster.Table Index Up-End": Value Change {
        w1229 = T11 {"CurrentImage"=refnum, "SavedImage"=refnum}  # Image Input Cluster
        # "Is no of rows > 1?"
        n370 = event-data() -> ()  [unwired: 1 in, 1 out]
        n371 = Unbundle By Name(w1221) -> ("Big Table"=w1239:refnum<vi>, "Notes Table"=w1238:refnum<vi>)
        n372 = Array Size(array=w1222) -> (size(s)=w1234:i32[])
        n373 = Bundle By Name(cluster=w1229, "SavedImage"=w1228, "CurrentImage"=w1218) -> (w1227:T11)
        n374 = Index Array(array=w1234, index=0) -> (element=w1232:i32)
        n375 = Build Array(w1239, w1238) -> (w1235:refnum<vi>[])
        n376 = Greater?(x=w1232, y=1) -> (0:w1231:bool)
        n377 = case shown="False" w1231 {
          tunnel: w1237 -> [w1246 w1261]
          tunnel: w1236 -> [w1245 w1260]
          tunnel: w1235 -> [_ w1257]
          tunnel: [w1245 w1251] -> w1223
          tunnel: [w1246 w1252] -> w1225
          tunnel: w1222 -> [_ w1250]
          tunnel: w1227 -> [w1244 w1248]
          tunnel: [w1243 w1247] -> w1219
          frame False {
            n378 = Unbundle By Name(w1244) -> ("SavedImage"=w1243:T7)
          }
          frame True {
            w1251 = 0
            n379 = call "FormatTableStyle.vi"("Format Command"=FormatTableStyle_Commands."Uncolour Row", "Error In"=w1261, "Row Index"=w1260, "Table reference Array"=w1257) -> ("Error Out"=w1262:errorcluster)  [unwired: 7 in]
            n380 = call "FormatTableStyle.vi"("Format Command"=FormatTableStyle_Commands."Colour Row", "Error In"=w1262, "Row Index"=w1251, "Table reference Array"=w1257) -> ("Error Out"=w1259:errorcluster)  [unwired: 7 in]
            n381 = call "FormatTableStyle.vi"("Format Command"=FormatTableStyle_Commands."UpdateVisibleRows", "Error In"=w1259, "Row Index"=w1251, "Table reference Array"=w1257) -> ("Error Out"=w1249:errorcluster)  [unwired: 7 in]
            n382 = Index Array(array=w1250, index (row)=w1251, index (col)=8 ("disabled index (col)")) -> (element=w1255:string)
            n383 = String To Path(string=w1255) -> (path=w1253:path)
            n384 = call "ImageIO.vi"("Pos_ImageIO_commands"=ImageIO_commands."ReadImage", "Error In"=w1249, "Image File Path"=w1253, "ImageCluster IN"=w1248) -> ("Error Out"=w1252:errorcluster, "Saved Image OUT"=w1247:T7)  [unwired: 5 in, 1 out]
          }
        }
        n385 = call "GenerateDisplayData.vi"("Index"=w1223, "Error In"=w1225, "UI Controls Refnum"=w1221, "2D Data IN"=w1222) -> ("Error Out"=w1224:errorcluster, "Plot Data OUT"=w1220:cluster{dbl[], dbl[]}[])  [unwired: 4 in, 2 out]
      }
      event "Table Navigation Cluster.Table Index Up": Value Change {
        w1277 = T11 {"CurrentImage"=refnum, "SavedImage"=refnum}  # Image Input Cluster
        n386 = event-data() -> ()  [unwired: 1 in, 1 out]
        n387 = Bundle By Name(cluster=w1277, "SavedImage"=w1276, "CurrentImage"=w1275) -> (w1274:T11)
        n388 = Unbundle By Name(w1267) -> ("Big Table"=w1282:refnum<vi>, "Notes Table"=w1281:refnum<vi>)
        n389 = Build Array(w1282, w1281) -> (w1280:refnum<vi>[])
        n390 = Greater Than 0?(x=w1278) -> (x > 0?=w1283:bool)
        n391 = case shown="False" w1283 {
          tunnel: w1278 -> [w1290 w1308]
          tunnel: [w1290 w1292] -> w1269
          tunnel: w1280 -> [_ w1301]
          tunnel: w1279 -> [w1289 w1307]
          tunnel: [w1289 w1296] -> w1271
          tunnel: w1274 -> [w1288 w1294]
          tunnel: w1268 -> [_ w1293]
          tunnel: [w1287 w1291] -> w1273
          frame False {
            n392 = Unbundle By Name(w1288) -> ("SavedImage"=w1287:T7)
          }
          frame True {
            n393 = call "FormatTableStyle.vi"("Format Command"=FormatTableStyle_Commands."Uncolour Row", "Error In"=w1307, "Row Index"=w1308, "Table reference Array"=w1301) -> ("Error Out"=w1306:errorcluster)  [unwired: 7 in]
            n394 = Decrement(x=w1308) -> (x-1=w1292:i32)
            n395 = call "FormatTableStyle.vi"("Format Command"=FormatTableStyle_Commands."Colour Row", "Error In"=w1306, "Row Index"=w1292, "Table reference Array"=w1301) -> ("Error Out"=w1303:errorcluster)  [unwired: 7 in]
            n396 = call "FormatTableStyle.vi"("Format Command"=FormatTableStyle_Commands."UpdateVisibleRows", "Error In"=w1303, "Row Index"=w1292, "Table reference Array"=w1301) -> ("Error Out"=w1295:errorcluster)  [unwired: 7 in]
            n397 = Index Array(array=w1293, index (row)=w1292, index (col)=8 ("disabled index (col)")) -> (element=w1299:string)
            n398 = String To Path(string=w1299) -> (path=w1297:path)
            n399 = call "ImageIO.vi"("Pos_ImageIO_commands"=ImageIO_commands."ReadImage", "Error In"=w1295, "Image File Path"=w1297, "ImageCluster IN"=w1294) -> ("Error Out"=w1296:errorcluster, "Saved Image OUT"=w1291:T7)  [unwired: 5 in, 1 out]
          }
        }
        n400 = call "GenerateDisplayData.vi"("Index"=w1269, "Error In"=w1271, "UI Controls Refnum"=w1267, "2D Data IN"=w1268) -> ("Error Out"=w1270:errorcluster, "Plot Data OUT"=w1266:cluster{dbl[], dbl[]}[])  [unwired: 4 in, 2 out]
      }
      event Value Change {
        # "Typecast to int to make it compatible\nwith both tab types (galvo and reso)"
        # "On user selecting a different channel,\nset the channel no variable to trigger\nthe user event case which refreshes\ncurrent data"
        n401 = event-data() -> ("NewVal"=w1325:T5)  [unwired: 1 in]
        n402 = call "Chnl_2_tab.vi"("Command"=Chnl_2_tab_Commands."ChannelToTab", "Error In"=w1327, "Channel IN"=w1325) -> ("Error Out"=w1326:errorcluster, "Tab Out"=w1316:T16)  [unwired: 6 in, 1 out]
        n403 = Type Cast(type=0 ("x-y 2"), x=w1316) -> (*(type *) &x=w1309:i32)
        n404 = Increment(x=w1309) -> (x+1=w1310:i32)
        n405 = Build Array("MAIN Image panels " ("Variable Name in"), "MAIN Image panels reso " ("Variable Name in")) -> (w1319:string[])
        n406 = for {
          tunnel: w1326 -> [w1337]
          tunnel: w1309 -> [w1336]
          tunnel: [w1335] -> w1314
          tunnel: w1319 -> [w1334] mode=indexing
          n407 = call "GFG_core.vi"("Variable Name in"=w1334, "Variant in"=w1336, "error in (no error)"=w1337, "Action"=enum16{"Init", "Set", "Get"}."Set") -> ("error out"=w1335:errorcluster)  [unwired: 9 in, 6 out]
        }
        n408 = call "GFG_core.vi"("Variable Name in"="channel.no", "Variant in"=w1310, "error in (no error)"=w1314, "Action"=enum16{"Init", "Set", "Get"}."Set") -> ("error out"=w1313:errorcluster)  [unwired: 9 in, 6 out]
      }
      event "step.size.xy 2": Value Change {
        n409 = event-data() -> ("NewVal"=w1349:u16)  [unwired: 1 in]
        n410 = To Variant(anything=w1349) -> (Variant=w1348:variant)
        n411 = call "GFG_core.vi"("Variable Name in"="step.size.xy", "Variant in"=w1348, "error in (no error)"=w1346, "Action"=enum16{"Init", "Set", "Get"}."Set") -> ("error out"=w1345:errorcluster)  [unwired: 9 in, 6 out]
      }
      event "FOCUS2": Value Change {
        n412 = event-data() -> ("NewVal"=w1360:bool)  [unwired: 1 in]
        n413 = To Variant(anything=w1360) -> (Variant=w1361:variant)
        n414 = call "GFGfpRefGet.vi"("Variable Name in"="FOCUS") -> ("output cluster"=w1363:T21)  [unwired: 9 in, 1 out]
        n415 = Unbundle By Name(w1363) -> ("BooleanRef"=w1362:refnum<vi>)
        n416 = property class="Bool"(reference=w1362, error in=w1359, "Val(Sgnl)"=w1361) -> (reference out=w1357:refnum<vi>, error out=w1358:errorcluster)
        n417 = Close Reference(reference=w1357, error in (no error)=w1358) -> (error out=w1356:errorcluster)
      }
      event Key Down {
        w1387 = T11 {"CurrentImage"=refnum, "SavedImage"=refnum}  # Image Input Cluster
        n418 = event-data() -> ("VKey"=w1388:T23)  [unwired: 1 in]
        n419 = Bundle By Name(cluster=w1387, "CurrentImage"=w1386, "SavedImage"=w1382) -> (w1385:T11)
        n420 = case shown="\"ASCII\", Default" w1388 {
          tunnel: w1379 -> [_ w1403 w1408 w1418 w1426]
          tunnel: w1385 -> [_ w1402 w1407 w1417 w1425]
          tunnel: w1378 -> [_ w1401 w1406 w1416 w1424]
          tunnel: w1384 -> [w1393 w1400 w1411 w1419 w1427]
          tunnel: w1383 -> [w1394 w1399 w1409 w1412 w1422]
          tunnel: [w1395 w1398 w1405 w1413 w1421] -> w1381
          tunnel: [w1394 w1397 w1404 w1414 w1420] -> w1377
          tunnel: [w1393 w1396 w1410 w1415 w1423] -> w1380
          tunnel: w1382 -> [w1395 _ _ _ _]
          frame "ASCII", Default {
          }
          frame "Down", "PageDown" {
            n421 = call "Table Index Down.vi"("Table Index IN"=w1399, "error in (no error)"=w1400, "UI Controls Refnum"=w1401, "Image cluster"=w1402, "Formatted Table Data"=w1403) -> ("error out"=w1396:errorcluster, "Table Index OUT"=w1397:i32, "Saved Image OUT"=w1398:T7)  [unwired: 4 in]
          }
          frame "End" {
            n422 = call "Table Index Down_End.vi"("Table Index IN"=w1409, "error in (no error)"=w1411, "UI Controls Refnum"=w1406, "Image cluster"=w1407, "Formatted Table Data"=w1408) -> ("error out"=w1410:errorcluster, "Table Index OUT"=w1404:i32, "Saved Image OUT"=w1405:T7)  [unwired: 4 in]
          }
          frame "Home" {
            n423 = call "Table Index Up_End.vi"("Table Index IN"=w1412, "error in (no error)"=w1419, "UI Controls Refnum"=w1416, "Image cluster"=w1417, "Formatted Table Data"=w1418) -> ("error out"=w1415:errorcluster, "Table Index OUT"=w1414:i32, "Saved Image OUT"=w1413:T7)  [unwired: 4 in]
          }
          frame "Up", "PageUp" {
            n424 = call "Table Index Up.vi"("Table Index IN"=w1422, "error in (no error)"=w1427, "UI Controls Refnum"=w1424, "Image cluster"=w1425, "Formatted Table Data"=w1426) -> ("error out"=w1423:errorcluster, "Table Index OUT"=w1420:i32, "Saved Image OUT"=w1421:T7)  [unwired: 4 in]
          }
        }
        n425 = call "GenerateDisplayData.vi"("Index"=w1377, "Error In"=w1380, "UI Controls Refnum"=w1378, "2D Data IN"=w1379) -> ("Error Out"=w1376:errorcluster, "Plot Data OUT"=w1375:cluster{dbl[], dbl[]}[])  [unwired: 4 in, 2 out]
      }
      event "Vert_Cluster.GO TO": Value Change {
        # "Set the GFG with the values of\nX, Y and Z in the table"
        n426 = event-data() -> ()  [unwired: 1 in, 1 out]
        n427 = Index Array(array=w1443, index (row) #1=w1440, index (col) #1=0 ("disabled index (col)"), index (row) #2=w1440, index (col) #2=1 ("index (row)"), index (row) #3=w1440, index (col) #3=2 ("disabled index (col)")) -> (element #1=w1438:string, element #2=w1437:string, element #3=w1436:string)
        n428 = Fract/Exp String To Number(string=w1438) -> (number=w1434:dbl)  [unwired: 3 in, 1 out]
        n429 = Fract/Exp String To Number(string=w1437) -> (number=w1433:dbl)  [unwired: 3 in, 1 out]
        n430 = Fract/Exp String To Number(string=w1436) -> (number=w1432:dbl)  [unwired: 3 in, 1 out]
        n431 = Bundle By Name(cluster=T17 {"moveXabs"=0.0, "moveYabs"=0.0, "moveZabs"=0.0} ("output cluster"), "moveXabs"=w1434, "moveYabs"=w1433, "moveZabs"=w1432) -> (w1429:T17)
        n432 = call "GFG_core.vi"("Variable Name in"="moveXYZabs", "Variant in"=w1429, "Action"=enum16{"Init", "Set", "Get"}."Set") -> ()  [unwired: 10 in, 7 out]
        n433 = disable-structure shown="Enabled" {
          disable-tunnel: w1434 -> [w1454 _]
          disable-tunnel: w1433 -> [w1453 _]
          disable-tunnel: w1432 -> [w1452 _]
          frame Disabled {
            w1455 = enum16{"Init", "Set", "Get"}."Set" ("Action")
            n434 = call "GFG_core.vi"("Variable Name in"="setY", "Variant in"=w1453, "Action"=w1455) -> ()  [unwired: 10 in, 7 out]
            n435 = call "GFG_core.vi"("Variable Name in"="setZ", "Variant in"=w1452, "Action"=w1455) -> ()  [unwired: 10 in, 7 out]
            n436 = call "GFG_core.vi"("Variable Name in"="setX", "Variant in"=w1454, "Action"=w1455) -> ()  [unwired: 10 in, 7 out]
          }
          frame Enabled {
          }
        }
      }
      event "step.size.z 2": Value Change {
        n437 = event-data() -> ("NewVal"=w1469:u16)  [unwired: 1 in]
        n438 = To Variant(anything=w1469) -> (Variant=w1468:variant)
        n439 = call "GFG_core.vi"("Variable Name in"="step.size.z", "Variant in"=w1468, "error in (no error)"=w1466, "Action"=enum16{"Init", "Set", "Get"}."Set") -> ("error out"=w1465:errorcluster)  [unwired: 9 in, 6 out]
      }
      event Value Change {
        # "Hide FP on user selection"
        n440 = event-data() -> ("NewVal"=w1482:T2)  [unwired: 1 in]
        n441 = case shown="False" w1482 {
          tunnel: [w1489 w1502] -> w1487
          tunnel: w1483 -> [w1491 w1502]
          frame False {
            n442 = control-ref of="This VI"() -> (w1501:refnum<vi>)
            n443 = invoke class="VI" method="FP.Close"(reference=w1501, error in=w1491) -> (reference out=w1499:refnum<vi>, error out=w1500:errorcluster)  [unwired: 1 in, 1 out]
            n444 = Close Reference(reference=w1499, error in (no error)=w1500) -> (error out=w1492:errorcluster)
            n445 = call "GFGfpRefGet.vi"("error in (no error)"=w1492, "Variable Name in"="PositionSaveButton") -> ("error out"=w1496:errorcluster, "output cluster"=w1497:T21)  [unwired: 8 in]
            n446 = Unbundle By Name(w1497) -> ("BooleanRef"=w1495:refnum<vi>)
            n447 = property class="Bool"(reference=w1495, error in=w1496, "Value"=FALSE) -> (reference out=w1493:refnum<vi>, error out=w1494:errorcluster)
            n448 = Close Reference(reference=w1493, error in (no error)=w1494) -> (error out=w1489:errorcluster)
          }
          frame True {
          }
        }
      }
    }
    "XY Graph" <- w93
    "posY 2" <- w103
    "posX 2" <- w94
    "posZ 2" <- w102
    "Current Image" <- w88
    "File Path" <- w95
    n449 = flat-sequence {
      frame #0 {
      }
    }
    n450 = Merge Errors(w82, w92) -> (w91:errorcluster)
    n451 = Bundle By Name(cluster=T11 {"CurrentImage"=refnum, "SavedImage"=refnum} ("Image Input Cluster"), "CurrentImage"=w88, "SavedImage"=w87) -> (w86:T11)
    n452 = Unbundle By Name(w91) -> ("status"=w112:bool)
    n453 = call "ImageOverlay.vi"("RGB_Image"=w84, "Error In"=w82, "Overlay?"="Overlay", "UI Controls Refnum"=w90, "Image Input Cluster"=w86) -> ("Error Out"=w81:errorcluster, "Saved Image"=→"Saved Image":T7)  [unwired: 5 in]
    n454 = Or(x=w112, y=w113) -> (x .or. y?=w111:bool)
  }
  n455 = Unregister For Events(event registration refnum=w54, error in=w24) -> (error out=w61:errorcluster)
  n456 = call <vilib>:"Simple Error Handler.vi"("error in (no error)"=w61) -> ("error out"=w25:errorcluster)  [unwired: 4 in, 4 out]
  n457 = call <vilib>:"Clear Errors.vi"("error in (no error)"=w25) -> ("error out"=w5:errorcluster)  [unwired: 6 in]
  n458 = call "IMAQ Dispose"("Image"=w3, "error in (no error)"=w5) -> ("error out"=w1:errorcluster)  [unwired: 4 in]
  n459 = call "IMAQ Dispose"("Image"=w2, "error in (no error)"=w1) -> ("error out"=w4:errorcluster)  [unwired: 4 in]
  n460 = call "PositionSaveFGV.vi"("PositionSave Commands"=PositionSaveFGVCommands."Shutdown and Cleanup", "Error In"=w4) -> ()  [unwired: 5 in, 5 out]
